vi "main.vi"() -> ()   [LabVIEW 2018]
uses:
  #include/Global_usbComm.vi
  <vilib>/Utility/file.llb/Read Delimited Spreadsheet (string).vi
panel:
  out "negative incline":dbl
  out "tabletType":string
  out "audioType":string
  out "Display":string
  out "TV":string
  out "decimal integer string":string
  out "device":u32
  out "FAN":string
  out "fanType":string
  out "upperLimit":dbl
  out "lowerLimit":dbl
  out "MAX":dbl
  out "upper":dbl
  out "middle":dbl
  out "lower":dbl
  out "minMax":dbl
  out "USB":string
  out "refnum out":refnum<file>
  in  "Tab Control":T1(tab)
  out "Welcome to Console Test":picture
  out "Version":string[][](array[string])
  in  "User Name":string
  out "Console Name":string
  out "Console Number":string
  in  "Work Station":string
  in  "Vendor Name":string
  in  "Vendor Number":string
  in  "EQF1259 com port":refnum<visa-resource-name>
  out "Firmware Reference":string
  out "Initialize Test":string
  out "Config and Fixture Setup":string
  in  "scanSerial":string="387495-JJ02Y101637"
  out "resultSerial":bool
  out "PartNumber":string
  out "COSMETIC-3, 4":string
  in  "Cos0":bool
  in  "Cos1":bool
  in  "Con0":bool
  in  "Con1":bool
  out "FIXTURE_SETUP-1":string
  out "Connection":picture
  out "Voltage":string
  out "Power On":cluster{dbl, dbl}(graph)
  out "Current":string
  out "POWER_UP-5, 6":string
  in  "Pow0":bool
  in  "Pow1":bool
  out "PowerOn":bool
  out "CurrentOn":bool
  out "BLE_SETUP-2":string
  out "BLE_CONNECT-7":string
  in  "BLE1":bool
  in  "BLE0":bool
  in  "Cal1":bool
  in  "Cal0":bool
  in  "Dis1":bool
  in  "Dis0":bool
  in  "key1":bool
  in  "key0":bool
  out "MAINTENANCE MODE-8, 9, 10, 11":string
  in  "Enter Firmware":string
  in  "E-Stop":bool
  out "MPH/KPH":string
  out "PWM":string
  out "FREQUENCY":string
  out "START":string
  out "MID":string
  out "SPEED TREADMILL":dbl(knob) scale=0.0..12.1
  out "MAX":string
  out "Smin":bool=TRUE
  out "Smid":bool=TRUE
  out "Smax":bool=TRUE
  out "PWM_RPM":string
  out "MaxSpeed Time (s)":dbl caption="Elapsed Time (s)"
  out "SPEED AEROBIC":dbl(knob) scale=0.0..25.0
  out "RPM AEROBIC":dbl(knob) scale=0.0..200.0
  in  "Tac0":bool
  in  "Tac1":bool
  in  "RES1":bool
  in  "RES0":bool
  out "overCurrent":bool
  out "RESISTANCE-15":string
  out "RESISTANCE/CURRENT":cluster{dbl, dbl}(graph)
  out "resistance result":bool
  out "ADC hi":bool=TRUE
  out "ADC mid":bool=TRUE
  out "ADC low":bool=TRUE
  out "ADC value":dbl
  out "current#":string
  out "BLE PULSE":u32(graph)
  in  "PUL1":bool
  in  "PUL0":bool
  out "Pulse#":u32
  out "PULSE-17":string
  out "FanCurrent":dbl(graph)
  in  "FAN1":bool
  in  "FAN0":bool
  out "Ifan":string
  out "limitFan":bool
  out "currentMaxFan":string
  out "FAN-18":string
  out "limitAudio":bool
  out "Iaudio":string
  out "AudioCurrent":dbl(graph)
  in  "AUD0":bool
  in  "AUD1":bool
  out "currentMaxAudio":string
  out "AUDIO-19":string
  in  "TV0":bool
  in  "TV1":bool
  out "TVCurrent":dbl(graph)
  out "Itv":string
  out "limitTV":bool
  out "currentMaxTV":string
  out "TV-20":string
  out "limitUSB":bool
  out "Iusb":string
  in  "USB1":bool
  in  "USB0":bool
  out "currentMaxUSB":string
  out "USBCurrent":dbl(graph)
  out "USB-16":string
  out "resultIncline":bool
  out "INCLINE":dbl(graph)
  in  "E-Stop/Incline":bool
  out "INCLINE-14":string
  out "inclineMax":dbl
  out "inclineMin":dbl
  out "inclineMid":dbl
  out "Imin":bool=TRUE
  out "Imid":bool=TRUE
  out "Imax":bool=TRUE
  out "Incline Time (s)":dbl caption="Elapsed Time (s)"
  out "limitCSafe":bool
  out "Icsafe":string
  in  "CSA1":bool
  in  "CSA0":bool
  out "currentMaxCSafe":string
  out "CSafeCurrent":dbl(graph)
  out "CSAFE-21":string
  out "limitWahoo":bool
  out "Iwahoo":string
  in  "WAH1":bool
  in  "WAH0":bool
  out "currentMaxWahoo":string
  out "WahooCurrent":dbl(graph)
  out "WAHOO-22":string
  in  "ANO0":bool
  in  "ANO1":bool
  out "Another":picture
  out "Failed":picture
  out "Test Log":string
  out "# of Failed Samples":i32
  out "# of Samples":i32
  out "Goodbye!":picture
  # "Scan Console Serial Number"
  # "Does Cosmetic Pass Inspection?"
  # "Is the console connected correctly?"
  # "Did Console Power ON?"
  # "Calibrate?"
  # "Display?"
  # "Keys?"
  # "Does Max Speed/RPM On Console Match Indicator?"
  # "Did Resistance Reach Max?"
  # "Does The Pulse# Match The Display?"
  # "Did The Fan Function Well?"
  # "Does Incline On Console Change?"
  # "Would You Like To Test Another Console?"
  # "Console Failed Test!"
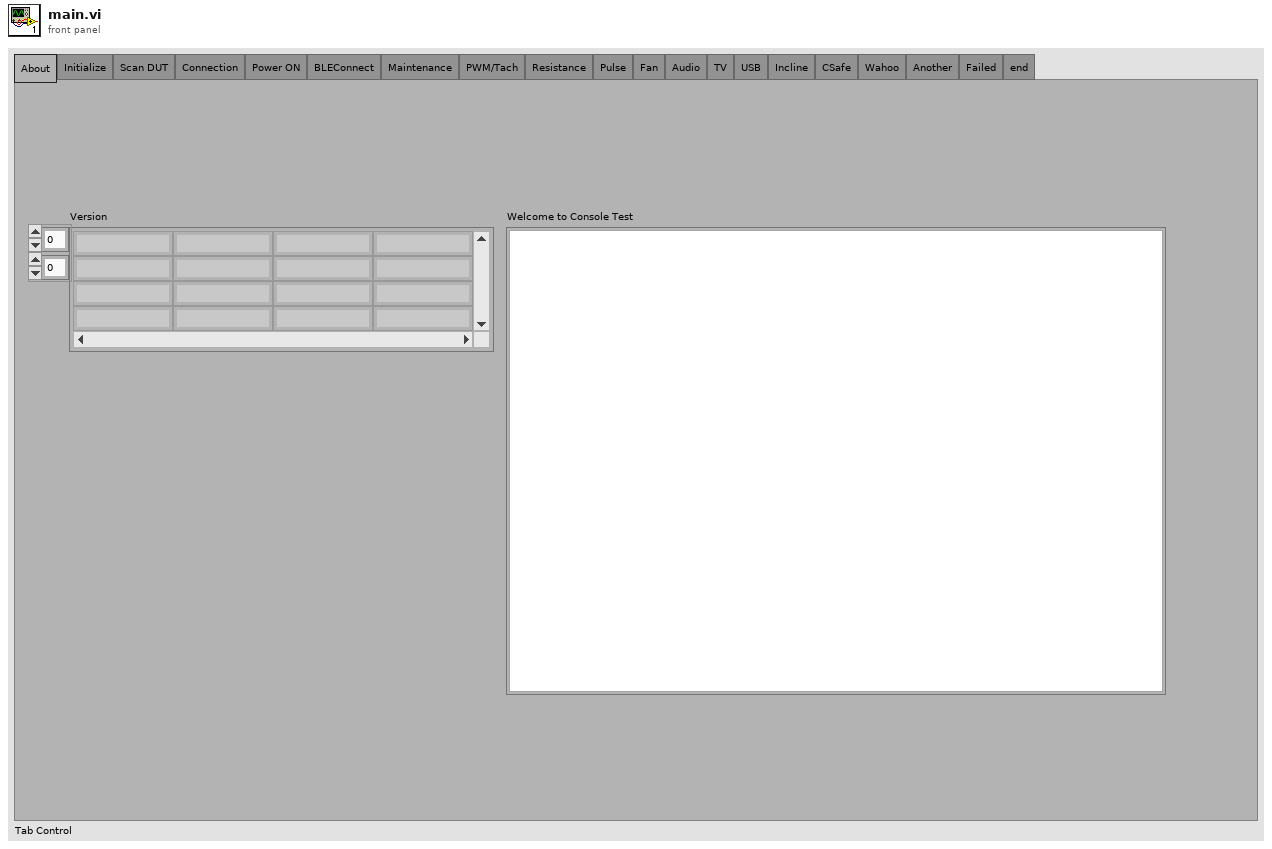
[diagram p1: front panel]
types:
  T1 = enum32{"About", "Initialize", "Scan DUT", "Connection", "Power ON", "BLEConnect", "Maintenance", "PWM/Tach", "Resistance", "Pulse", "Fan", "Audio", "TV", "USB", "Incline", "CSafe", "Wahoo", "Another", "Failed", "end"}
  T2 = enum16{"name", "number", "type", "ctlr/pwrbrd", "firmware", "mcu", "display"}
  T3 = enum16{"User", "Station", "Vendor", "Number", "Record"}
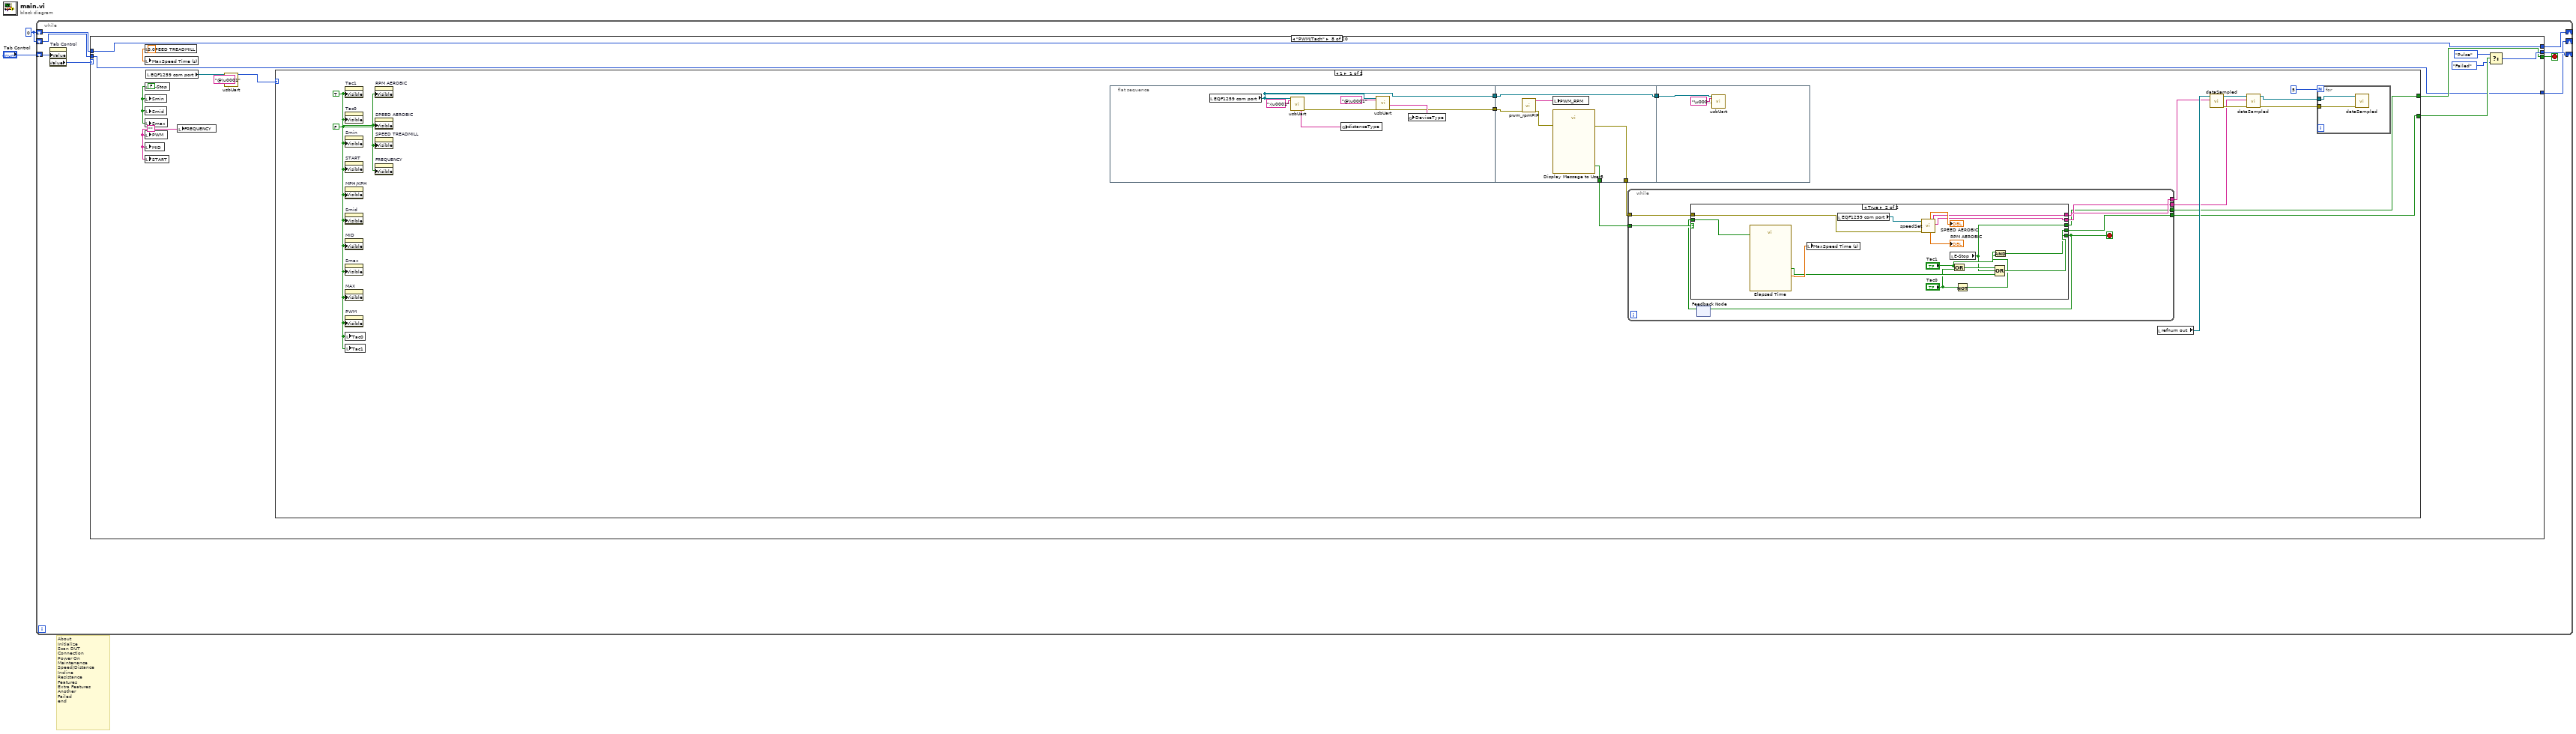
[diagram p0: block diagram]
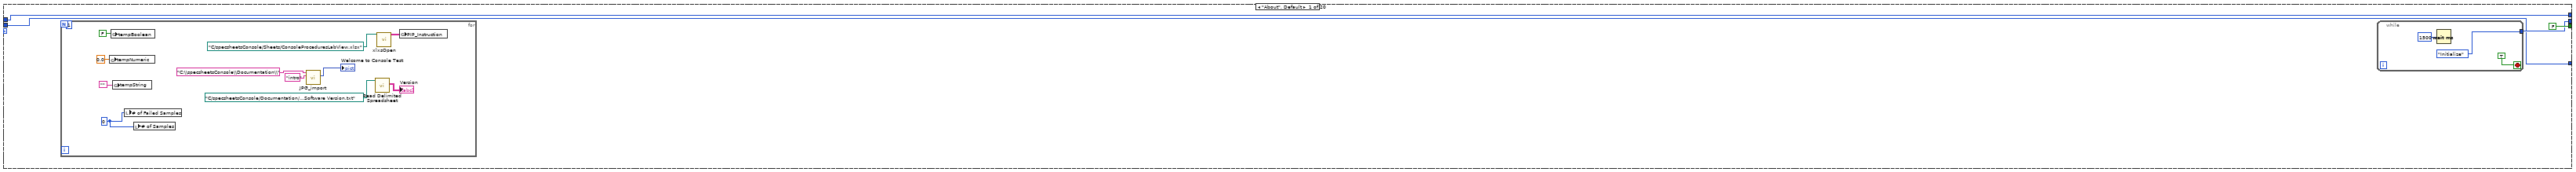
[diagram p2: hidden frame]
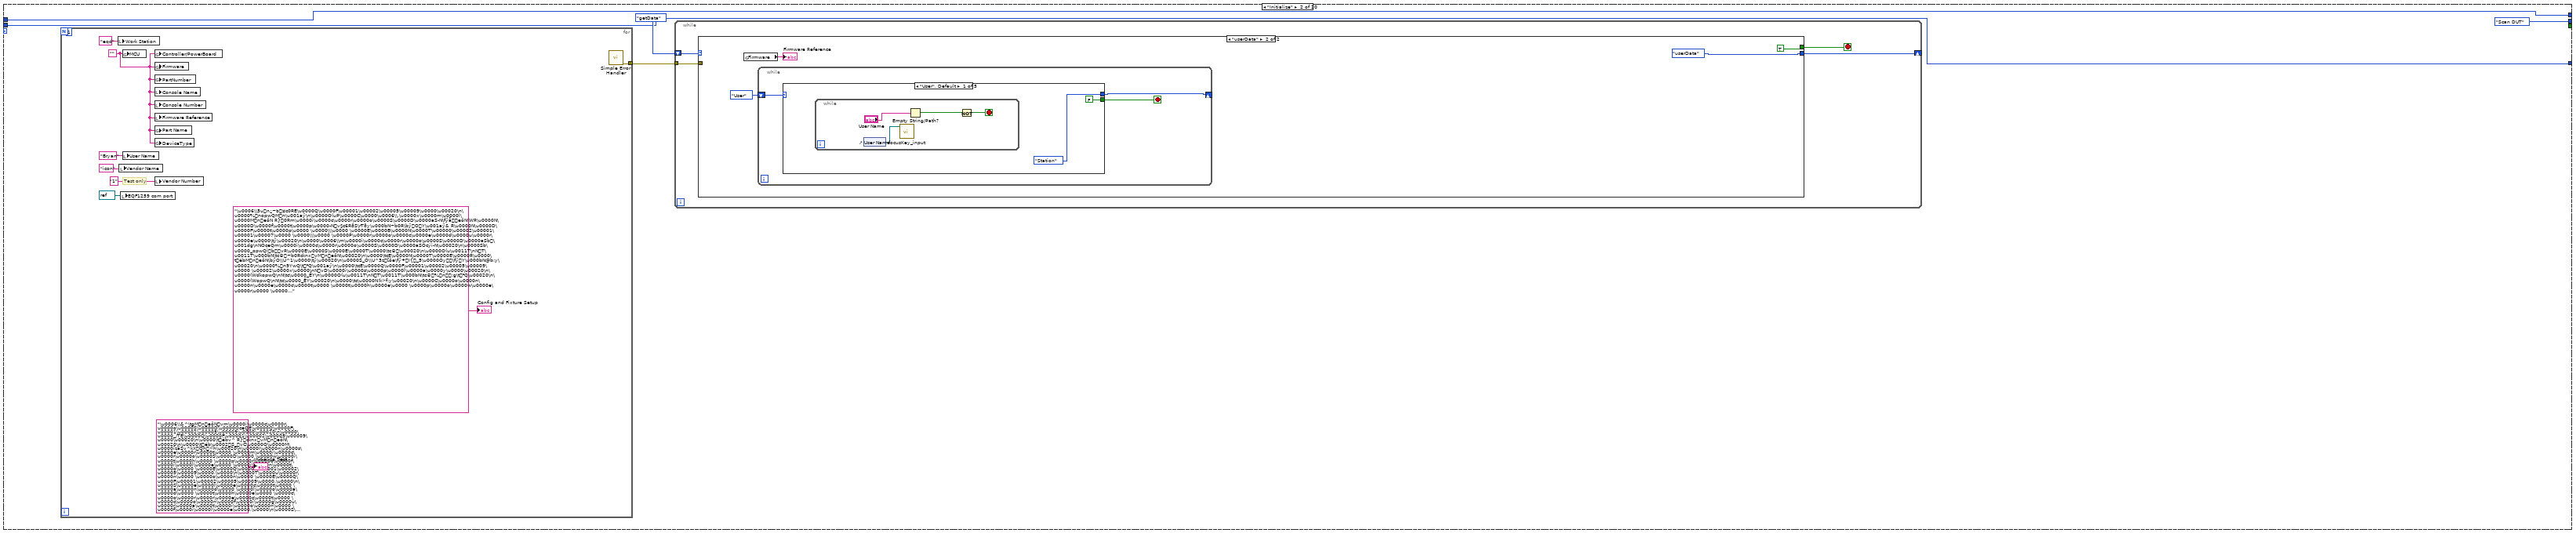
[diagram p3: hidden frame]
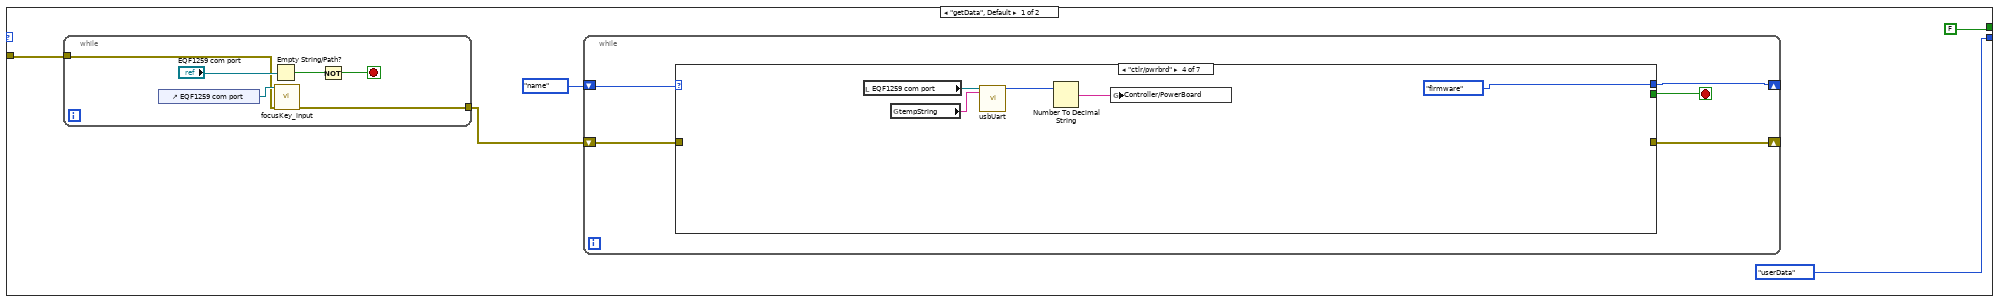
[diagram p4: hidden frame]
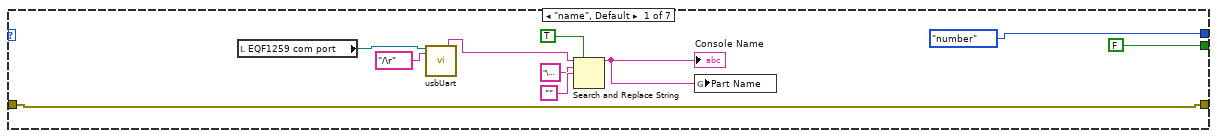
[diagram p5: hidden frame]
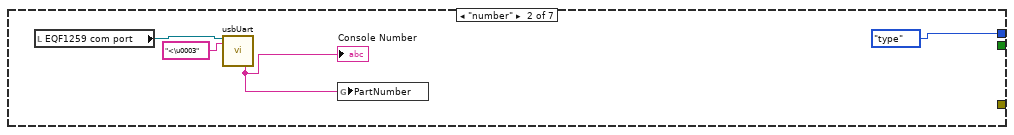
[diagram p6: hidden frame]
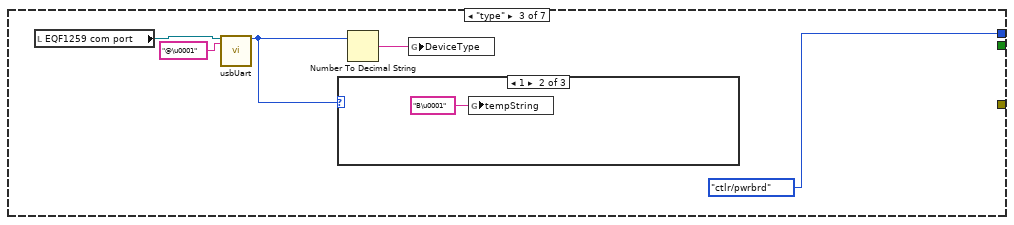
[diagram p7: hidden frame]
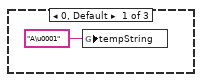
[diagram p8: hidden frame]
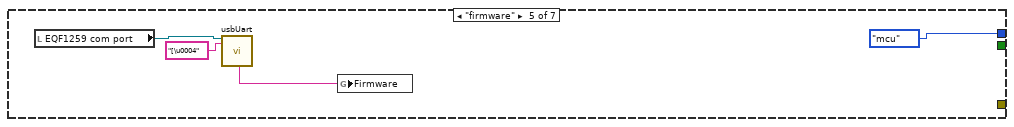
[diagram p10: hidden frame]
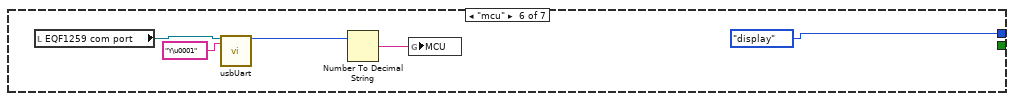
[diagram p11: hidden frame]
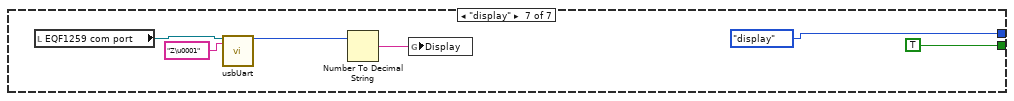
[diagram p12: hidden frame]
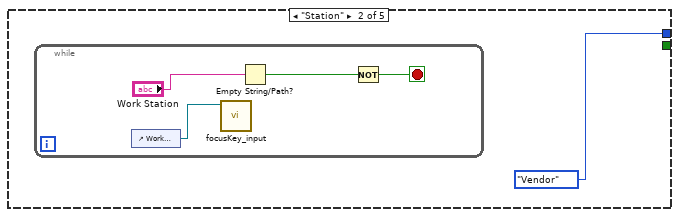
[diagram p13: hidden frame]
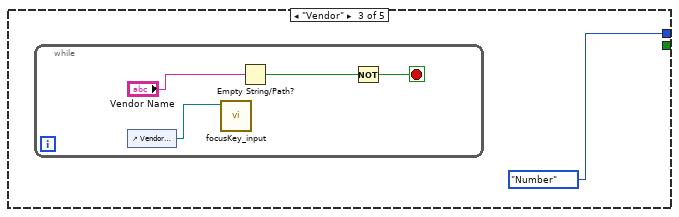
[diagram p14: hidden frame]
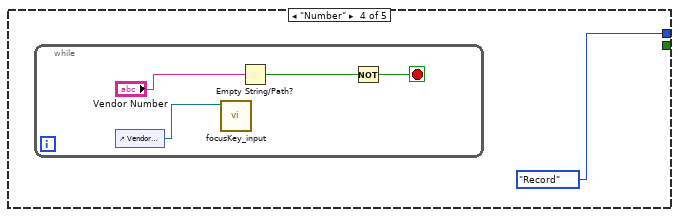
[diagram p15: hidden frame]
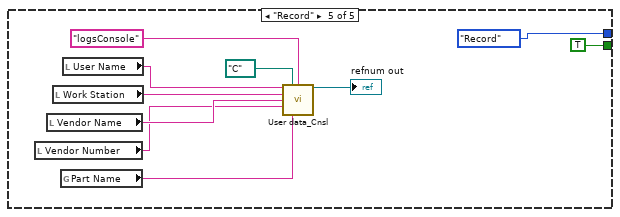
[diagram p16: hidden frame]
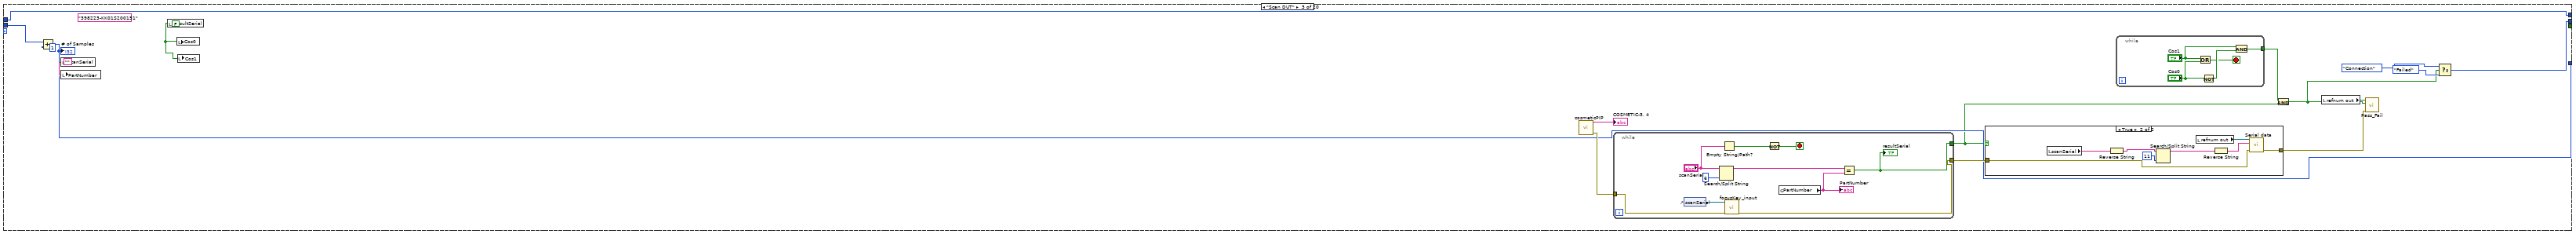
[diagram p17: hidden frame]
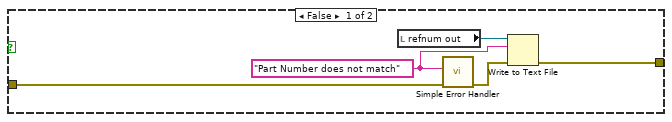
[diagram p18: hidden frame]
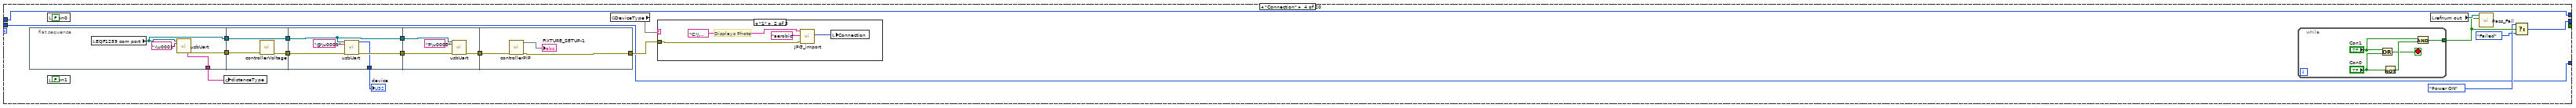
[diagram p19: hidden frame]
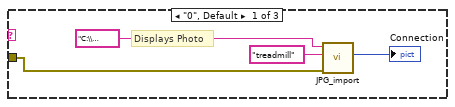
[diagram p20: hidden frame]
diagram:
  w1 = 0
  # "About\nInitialize\nScan DUT\nConnection\nPower On\nMaintenance\nSpeed/Distance\nIncline\nResistance\nFeatures\nExtra Features\nAnother\nFailed\nend"
  n1 = while {
    shift-right: [w9] -> _
    shift-left: "Tab Control" -> [w8]
    shift-right: [w4] -> _
    shift-left: w1 -> [w6]
    shift-right: [w3] -> _
    shift-left: w1 -> [w5]
    stop <- w10 stop-if-true
    n2 = property on="Tab Control" class="TabCtl (strict)"("Value"=w8) -> ("Value"=w7:T1)  [unwired: 2 in, 2 out]
    n3 = case shown="\"PWM/Tach\"" w7 {
      tunnel: [FALSE _ _ _ _ _ _ w444 w643 _ _ _ _ _ _ _ _ _ _ TRUE] -> w10
      tunnel: [w13 T1."Scan DUT" ("Tab Control") w152 w200 w258 w327 w363 w446 w645 w765 w901 w941 w1023 w1051 w1151 w1228 w1288 w1347 T1."Another" ("Tab Control") T1."end" ("Tab Control")] -> w9
      tunnel: w6 -> [w12 w31 w150 w190 w246 w323 w356 w435 w639 w756 w890 w922 w1000 w1043 w1140 w1218 w1277 w1336 w1354 w1368]
      tunnel: w5 -> [w11 w30 w148 w189 w245 w322 w355 w434 w638 w755 w889 w921 w999 w1042 w1139 w1217 w1276 w1335 w1356 w1367]
      tunnel: [w12 w31 w149 w190 w246 w323 w356 w435 w639 w756 w890 w922 w1000 w1043 w1140 w1218 w1277 w1336 w1354 w1368] -> w4
      tunnel: [w11 w30 w148 w189 w245 w322 w355 w434 w638 w755 w889 w921 w999 w1042 w1139 w1217 w1276 w1335 w1355 w1367] -> w3
      frame "About", Default {
        n4 = for {
          N: 1 -> [_]
          w16 = 0
          n5 = global write "Global_usbComm.vi" "tempNumeric"(0.0 ("tempNumeric")) -> ()
          n6 = global write "Global_usbComm.vi" "tempBoolean"(FALSE) -> ()
          n7 = global write "Global_usbComm.vi" "tempString"("" ("tempString")) -> ()
          n8 = local write "# of Failed Samples"(w16) -> ()
          n9 = local write "# of Samples"(w16) -> ()
          n10 = call "JPG_import.vi"("File name"="intro" ("Complete File path"), "File path"="C:\\specsheetsConsole\\Documentation\\" ("File name")) -> ("new picture"=→"Welcome to Console Test":picture)  [unwired: 7 in, 2 out]
          n11 = call-poly <vilib>:"Read Delimited Spreadsheet.vi"("file path (dialog if empty)"=path "C:/specsheetsConsole/Documentation/...Software Version.txt") -> ("all rows"=→"Version":string[][])  [unwired: 9 in, 5 out]
          n12 = call "xlxsOpen.vi"("PIP Instruction Path"=path "C:/specsheetsConsole/Sheets/ConsoleProceduresLabView.xlsx") -> ("Shared_strings"=w25:string[][])  [unwired: 10 in, 4 out]
          n13 = global write "Global_usbComm.vi" "PIP_Instruction"(w25) -> ()
        }
        n14 = while {
          tunnel: [T1."Initialize" ("Tab Control")] -> w13
          stop <- TRUE stop-if-true
          n15 = Wait (ms)(milliseconds to wait=u32 1500) -> ()  [unwired: 1 out]
        }
      }
      frame "Initialize" {
        n16 = for {
          N: 1 -> [_]
          tunnel: [w37] -> w33
          w43 = ""
          # "Test only"
          n17 = local write "Work Station"("eqd" ("Work Station")) -> ()
          n18 = local write "Vendor Name"("icon" ("Vendor Name")) -> ()
          n19 = local write "EQF1259 com port"(refnum<visa-resource-name> refnum ("VISA resource name")) -> ()
          n20 = global write "Global_usbComm.vi" "MCU"(w43) -> ()
          n21 = local write "User Name"("Bryan" ("User Name")) -> ()
          n22 = global write "Global_usbComm.vi" "Controller/PowerBoard"(w43) -> ()
          n23 = global write "Global_usbComm.vi" "Firmware"(w43) -> ()
          n24 = global write "Global_usbComm.vi" "PartNumber"(w43) -> ()
          n25 = local write "Console Name"(w43) -> ()
          n26 = local write "Console Number"(w43) -> ()
          n27 = local write "Firmware Reference"(w43) -> ()
          n28 = global write "Global_usbComm.vi" "Part Name"(w43) -> ()
          n29 = global write "Global_usbComm.vi" "DeviceType"(w43) -> ()
          n30 = local write "Vendor Number"("1" ("Vendor Number")) -> ()
          n31 = call <vilib>:"Simple Error Handler.vi"() -> ("error out"=w37:errorcluster)  [unwired: 5 in, 4 out]
          "Initialize Test" <- "\u0006\\&^\tgMneöNvm\u0000i\u0000c\u0000r\u0000o\u0000S\u0000D\u0000ÒceQE\u0000Q\u0000F\u00001\u00002\u00005\u00009\u0000\u00020\n\u0000\u0000_/TE\u0000Q\u0000F\u00001\u00002\u00005\u00009\u0000\u00020\n\u0000\tébv^ R}cknxvMneöN\u00020\n\u0000\téb\u0002S_vC\u0000O\u0000M\u0000ïzãSv^kXQh<h\u00020\n\u0000I\u0000n\u0000s\u0000e\u0000r\u0000t\u0000 \u0000m\u0000i\u0000c\u0000r\u0000o\u0000S\u0000D\u0000 \u0000w\u0000i\u0000t\u0000h\u0000 \u0000p\u0000r\u0000o\u0000f\u0000i\u0000l\u0000e\u0000 \u0000i\u0000n\u0000t\u0000o\u0000 \u0000E\u0000Q\u0000F\u00001\u00002\u00005\u00009\u0000.\u0000\n\u0000T\u0000u\u0000r\u0000n\u0000 \u0000o\u0000n\u0000 \u0000E\u0000Q\u0000F\u00001\u00002\u00005\u00009\u0000.\u0000\n\u0000S\u0000e\u0000l\u0000e\u0000c\u0000t\u0000 \u0000a\u0000n\u0000d\u0000 \u0000l\u0000o\u0000a\u0000d\u0000 \u0000t\u0000h\u0000e\u0000 \u0000c\u0000o\u0000r\u0000r\u0000e\u0000c\u0000t\u0000 \u0000c\u0000o\u0000n\u0000f\u0000i\u0000g\u0000u\u0000r\u0000a\u0000t\u0000i\u0000o\u0000n\u0000 \u0000f\u0000i\u0000l\u0000e\u0000.\u0000\n\u0000S\u0000e\u0000l\u0000e\u0000c\u0000t\u0000 \u0000t\u0000h\u0000e\u0000 \u0000p\u0000r\u0000o\u0000p\u0000e\u0000r\u0000 \u0000c\u0000o\u0000m\u0000 \u0000p\u0000o\u0000r\u0000t\u0000 \u0000a\u0000n\u0000d\u0000 \u0000c\u0000o\u0000m\u0000p\u0000l\u0000e\u0000t\u0000e\u0000 \u0000t\u0000h\u0000e\u0000 \u0000f\u0000o\u0000r\u0000m\u0000.\u0000"
          "Config and Fixture Setup" <- "\u0006\\5un¿~Þ¥c0RE\u0000Q\u0000F\u00001\u00002\u00005\u00009\u0000\u00020\n\u0000¾nopwQMn\u001aÿ\n\u0000O(uP\u0000C\u0000\u0006\\.\u0000x\u0000m\u0000l\u0000MneöN R}0Rm\u0000i\u0000c\u0000r\u0000o\u0000S\u0000D\u0000aS-N\fÿåeöN(WR\u0000N\u0000D\u0000f\u0000t\u0000p\u0000-Nv§c6RðS\rTðy\u000bN~b0R\bÿOY\u001aÿ& R\u0000N\u0000D\u0000F\u0000t\u0000p\u0000 \u0000\\\u0000 \u0000E\u0000B\u0000N\u0000T\u00000\u00002\u00001\u00001\u00007\u0000 \u0000\\\u0000 \u0000P\u0000r\u0000o\u0000c\u0000e\u0000d\u0000u\u0000r\u0000e\u0000\tÿ\u00020\n\u0000\u0006\\m\u0000i\u0000c\u0000r\u0000o\u0000S\u0000D\u0000aSb\u001dg\nNÒceQm\u0000i\u0000c\u0000r\u0000o\u0000S\u0000D\u0000aSÒcýi-N\u00020\n\u0000Sb\u0000_opwQÌbvR\u0000E\u0000S\u0000E\u0000T\u0000\tc®\u00020\n\u0000O(u\u0011T\nNT\u0011T\u000bN\tc®~b0RcknxvMneöN\u00020\n\u0000\tcE\u0000N\u0000T\u0000E\u0000R\u0000\tébMneöN\bÿO\\U^1\u0000\tÿ\u00020\n\u0000S_O\\U^3z[öe\fÿ÷I{_5\u0000Òy\fÿY\u000bN@b:y\u00020\n\u0000¾n9YwQ\t²Q\u001aÿ\n\u0000\tcE\u0000Q\u0000F\u00001\u00002\u00005\u00009\u0000 \u00002\u0000x\u0000\nNvD\u0000i\u0000s\u0000p\u0000l\u0000a\u0000y\u0000\u00020\n\u0000(WdkopwQ\nN\tc\u0000_ËY\n\u0000O(u\u0011T\nNT\u0011T\u000bN\tc®¾n:g\t²Q\u00020\n\u0000(WopwQ\nN\tc\u0000_ËY\u00020\n\u0000\tc\u0000N!k>f:y\u00020\n\u0000C\u0000o\u0000n\u0000n\u0000e\u0000c\u0000t\u0000 \u0000t\u0000h\u0000e\u0000 \u0000p\u0000o\u0000w\u0000e\u0000r\u0000 \u0000..."
        }
        n32 = while {
          shift-right: [w46] -> _
          shift-left: enum16{"getData", "userData"}."getData" -> [w48]
          tunnel: w33 -> [w45]
          stop <- w47 stop-if-true
          n33 = case shown="\"userData\"" w48 {
            tunnel: [FALSE TRUE] -> w47
            tunnel: [enum16{"getData", "userData"}."userData" enum16{"getData", "userData"}."userData"] -> w46
            tunnel: w45 -> [w49 _]
            frame "getData", Default {
              n34 = while {
                tunnel: [w55] -> w51
                tunnel: w49 -> [w54]
                stop <- w56 stop-if-true
                n35 = control-ref of="EQF1259 com port"() -> (w59:refnum<vi>)
                n36 = Empty String/Path?(string/path="EQF1259 com port") -> (empty?=w57:bool)
                n37 = call "focusKey_input.vi"("error in (no error)"=w54, "reference"=w59) -> ("error out"=w55:errorcluster)  [unwired: 9 in]
                n38 = Not(x=w57) -> (.not. x?=w56:bool)
              }
              n39 = while {
                shift-right: [w60] -> _
                shift-left: T2."name" -> [w64]
                shift-right: [w61] -> _
                shift-left: w51 -> [w62]
                stop <- w63 stop-if-true
                n40 = case shown="\"ctlr/pwrbrd\"" w64 {
                  tunnel: [FALSE _ _ _ _ _ TRUE] -> w63
                  tunnel: w62 -> [w71 _ _ _ _ _ _]
                  tunnel: [T2."number" T2."type" T2."ctlr/pwrbrd" T2."firmware" T2."mcu" T2."display" T2."display"] -> w60
                  tunnel: [w71 _ _ _ _ _ _] -> w61
                  frame "name", Default {
                    n41 = local read "EQF1259 com port"() -> (w72:refnum<visa-resource-name>)
                    n42 = call "usbUart.vi"("VISA resource name"=w72, "write buffer"="/\r" ("write buffer buffer")) -> ("valid byte"=w69:string)  [unwired: 2 in, 15 out]
                    n43 = Search and Replace String(replace all?=TRUE ("replace all? (F)"), input string=w69, search string="\u0000", replace string="") -> (result string=w66:string)  [unwired: 4 in, 3 out]
                    "Console Name" <- w66
                    n44 = global write "Global_usbComm.vi" "Part Name"(w66) -> ()
                  }
                  frame "number" {
                    n45 = local read "EQF1259 com port"() -> (w77:refnum<visa-resource-name>)
                    n46 = call "usbUart.vi"("VISA resource name"=w77, "write buffer"="<\u0003" ("write buffer buffer")) -> ("PartNumber"=w76:string)  [unwired: 2 in, 15 out]
                    "Console Number" <- w76
                    n47 = global write "Global_usbComm.vi" "PartNumber"(w76) -> ()
                  }
                  frame "type" {
                    n48 = local read "EQF1259 com port"() -> (w82:refnum<visa-resource-name>)
                    n49 = call "usbUart.vi"("VISA resource name"=w82, "write buffer"="@\u0001" ("write buffer buffer")) -> ("number[0]"=w81:u32)  [unwired: 2 in, 15 out]
                    n50 = case shown="1" w81 {
                      frame 0, Default {
                        n51 = global write "Global_usbComm.vi" "tempString"("A\u0001" ("write buffer buffer")) -> ()
                      }
                      frame 1 {
                        n52 = global write "Global_usbComm.vi" "tempString"("B\u0001" ("write buffer")) -> ()
                      }
                      frame 3 {
                        # "Rower_Basic"
                      }
                    }
                    n53 = Number To Decimal String(number=w81) -> (decimal integer string=w80:string)  [unwired: 1 in]
                    n54 = global write "Global_usbComm.vi" "DeviceType"(w80) -> ()
                  }
                  frame "ctlr/pwrbrd" {
                    n55 = local read "EQF1259 com port"() -> (w90:refnum<visa-resource-name>)
                    n56 = global read "Global_usbComm.vi" "tempString"() -> (w87:string)
                    n57 = call "usbUart.vi"("VISA resource name"=w90, "write buffer"=w87) -> ("number[0]"=w89:u32)  [unwired: 2 in, 15 out]
                    n58 = Number To Decimal String(number=w89) -> (decimal integer string=w88:string)  [unwired: 1 in]
                    n59 = global write "Global_usbComm.vi" "Controller/PowerBoard"(w88) -> ()
                  }
                  frame "firmware" {
                    n60 = local read "EQF1259 com port"() -> (w94:refnum<visa-resource-name>)
                    n61 = call "usbUart.vi"("VISA resource name"=w94, "write buffer"="[\u0004") -> ("BB FW"=w92:string)  [unwired: 2 in, 15 out]
                    n62 = global write "Global_usbComm.vi" "Firmware"(w92) -> ()
                  }
                  frame "mcu" {
                    n63 = local read "EQF1259 com port"() -> (w97:refnum<visa-resource-name>)
                    n64 = call "usbUart.vi"("VISA resource name"=w97, "write buffer"="Y\u0001") -> ("number[0]"=w99:u32)  [unwired: 2 in, 15 out]
                    n65 = Number To Decimal String(number=w99) -> (decimal integer string=w96:string)  [unwired: 1 in]
                    n66 = global write "Global_usbComm.vi" "MCU"(w96) -> ()
                  }
                  frame "display" {
                    n67 = local read "EQF1259 com port"() -> (w102:refnum<visa-resource-name>)
                    n68 = call "usbUart.vi"("VISA resource name"=w102, "write buffer"="Z\u0001") -> ("number[0]"=w105:u32)  [unwired: 2 in, 15 out]
                    n69 = Number To Decimal String(number=w105) -> (decimal integer string=w103:string)  [unwired: 1 in]
                    n70 = global write "Global_usbComm.vi" "Display"(w103) -> ()
                  }
                }
              }
            }
            frame "userData" {
              n71 = global read "Global_usbComm.vi" "Firmware"() -> (→"Firmware Reference":string)
              n72 = while {
                shift-right: [w110] -> _
                shift-left: T3."User" -> [w112]
                stop <- w111 stop-if-true
                n73 = case shown="\"User\", Default" w112 {
                  tunnel: [FALSE _ _ _ TRUE] -> w111
                  tunnel: [T3."Station" T3."Vendor" T3."Number" T3."Record" T3."Record"] -> w110
                  frame "User", Default {
                    n74 = while {
                      stop <- w116 stop-if-true
                      n75 = control-ref of="User Name"() -> (w115:refnum<vi>)
                      n76 = call "focusKey_input.vi"("reference"=w115) -> ()  [unwired: 10 in, 1 out]
                      n77 = Empty String/Path?(string/path="User Name") -> (empty?=w118:bool)
                      n78 = Not(x=w118) -> (.not. x?=w116:bool)
                    }
                  }
                  frame "Station" {
                    n79 = while {
                      stop <- w121 stop-if-true
                      n80 = control-ref of="Work Station"() -> (w120:refnum<vi>)
                      n81 = call "focusKey_input.vi"("reference"=w120) -> ()  [unwired: 10 in, 1 out]
                      n82 = Empty String/Path?(string/path="Work Station") -> (empty?=w123:bool)
                      n83 = Not(x=w123) -> (.not. x?=w121:bool)
                    }
                  }
                  frame "Vendor" {
                    n84 = while {
                      stop <- w126 stop-if-true
                      n85 = control-ref of="Vendor Name"() -> (w125:refnum<vi>)
                      n86 = call "focusKey_input.vi"("reference"=w125) -> ()  [unwired: 10 in, 1 out]
                      n87 = Empty String/Path?(string/path="Vendor Name") -> (empty?=w128:bool)
                      n88 = Not(x=w128) -> (.not. x?=w126:bool)
                    }
                  }
                  frame "Number" {
                    n89 = while {
                      stop <- w131 stop-if-true
                      n90 = control-ref of="Vendor Number"() -> (w130:refnum<vi>)
                      n91 = call "focusKey_input.vi"("reference"=w130) -> ()  [unwired: 10 in, 1 out]
                      n92 = Empty String/Path?(string/path="Vendor Number") -> (empty?=w133:bool)
                      n93 = Not(x=w133) -> (.not. x?=w131:bool)
                    }
                  }
                  frame "Record" {
                    n94 = local read "Vendor Number"() -> (w137:string)
                    n95 = local read "Vendor Name"() -> (w140:string)
                    n96 = local read "Work Station"() -> (w141:string)
                    n97 = global read "Global_usbComm.vi" "Part Name"() -> (w136:string)
                    n98 = local read "User Name"() -> (w142:string)
                    n99 = call "User data_Cnsl.vi"("Inspector"=w142, "base path"=path "C:/", "prompt (Create Folder)"="logsConsole", "Station"=w141, "Vendor"=w140, "Number"=w137, "file name"=w136) -> ("refnum out"=→"refnum out":refnum<file>)  [unwired: 7 in, 1 out]
                  }
                }
              }
            }
          }
        }
      }
      frame "Scan DUT" {
        (unwired) "398223-KK01S200151"
        w144 = FALSE
        w155 = ""
        n100 = Add(x=w150, y=1) -> (x+y=w149:i32)
        "# of Samples" <- w149
        n101 = local write "scanSerial"(w155) -> ()
        n102 = local write "PartNumber"(w155) -> ()
        n103 = local write "resultSerial"(w144) -> ()
        n104 = local write "Cos0"(w144) -> ()
        n105 = local write "Cos1"(w144) -> ()
        n106 = call "cosmeticPIP.vi"() -> ("error out"=w156:errorcluster, "COSMETIC-3, 4"=→"COSMETIC-3, 4":string)  [unwired: 10 in]
        n107 = while {
          tunnel: [w186] -> w160
          tunnel: [w180] -> w145
          tunnel: w156 -> [w179]
          stop <- w187 stop-if-true
          n108 = control-ref of="scanSerial"() -> (w185:refnum<vi>)
          n109 = Search/Split String(string="scanSerial", offset (0)=6) -> (substring before match=w184:string)  [unwired: 1 in, 2 out]
          n110 = Empty String/Path?(string/path="scanSerial") -> (empty?=w188:bool)
          n111 = call "focusKey_input.vi"("error in (no error)"=w179, "reference"=w185) -> ("error out"=w186:errorcluster)  [unwired: 9 in]
          n112 = Not(x=w188) -> (.not. x?=w187:bool)
          n113 = global read "Global_usbComm.vi" "PartNumber"() -> (w183:string)
          "PartNumber" <- w183
          n114 = Equal?(x=w184, y=w183) -> (x = y?=w180:bool)
          "resultSerial" <- w180
        }
        n115 = case shown="True" w145 {
          tunnel: w160 -> [w166 w171]
          tunnel: [w167 w172] -> w158
          frame False {
            w169 = "Part Number does not match" ("error source (\" \")")
            n116 = local read "refnum out"() -> (w168:refnum<file>)
            n117 = call <vilib>:"Simple Error Handler.vi"("error source (\" \")"=w169, "error in (no error)"=w166) -> ("error out"=w170:errorcluster)  [unwired: 3 in, 4 out]
            n118 = Write to Text File(file (use dialog)=w168, text=w169, error in=w170) -> (error out=w167:errorcluster)  [unwired: 1 in, 2 out]
          }
          frame True {
            n119 = local read "scanSerial"() -> (w175:string)
            n120 = Reverse String(1:w175) -> (0:w177:string)
            n121 = Search/Split String(string=w177, offset (0)=11) -> (substring before match=w178:string)  [unwired: 1 in, 2 out]
            n122 = local read "refnum out"() -> (w173:refnum<file>)
            n123 = Reverse String(1:w178) -> (0:w174:string)
            n124 = call "Serial data.vi"("error in"=w171, "Serial Number"=w174, "refnum in"=w173) -> ("error out"=w172:errorcluster)  [unwired: 7 in, 1 out]
          }
        }
        n125 = while {
          tunnel: [w161] -> w146
          stop <- w164 stop-if-true
          n126 = Or(x="Cos1", y="Cos0") -> (x .or. y?=w164:bool)
          n127 = Not(x="Cos0") -> (.not. x?=w165:bool)
          n128 = And(x="Cos1", y=w165) -> (x .and. y?=w161:bool)
        }
        n129 = And(x=w146, y=w145) -> (x .and. y?=w147:bool)
        n130 = local read "refnum out"() -> (w159:refnum<file>)
        n131 = call "Pass_Fail.vi"("error in (no error)"=w158, "OK"=w147, "Byte Stream File in"=w159) -> ()  [unwired: 7 in, 2 out]
        n132 = Select(t=T1."Connection" ("Tab Control"), s=w147, f=T1."Failed" ("Tab Control")) -> (s? t:f=w152:T1)
      }
      frame "Connection" {
        n133 = flat-sequence {
          tunnel: [w211] -> w204
          tunnel: [w210] -> w199
          tunnel: [w209] -> w197
          tunnel: w199 -> [w214]
          tunnel: [w213] -> w198
          tunnel: w197 -> [w215]
          tunnel: [w215] -> w196
          tunnel: w198 -> [w219]
          tunnel: w196 -> [w217]
          tunnel: [w218] -> w194
          tunnel: [w217] -> w192
          tunnel: [w216] -> w191
          tunnel: w194 -> [w224]
          tunnel: [w223] -> w193
          tunnel: w192 -> [w222]
          tunnel: w193 -> [w226]
          tunnel: [w225] -> w195
          frame #0 {
            n134 = local read "EQF1259 com port"() -> (w209:refnum<visa-resource-name>)
            n135 = call "usbUart.vi"("VISA resource name"=w209, "write buffer"="›\u0001") -> ("PartNumber"=w211:string, "error out"=w210:errorcluster)  [unwired: 2 in, 14 out]
          }
          frame #1 {
            n136 = call "controllerVoltage.vi"("error in (no error)"=w214) -> ("error out"=w213:errorcluster)  [unwired: 10 in]
          }
          frame #2 {
            n137 = call "usbUart.vi"("VISA resource name"=w217, "write buffer"="@\u0001", "error in (no error)"=w219) -> ("number[0]"=w216:u32, "error out"=w218:errorcluster)  [unwired: 1 in, 14 out]
          }
          frame #3 {
            n138 = call "usbUart.vi"("VISA resource name"=w222, "write buffer"="P\u0002", "error in (no error)"=w224) -> ("error out"=w223:errorcluster)  [unwired: 1 in, 15 out]
          }
          frame #4 {
            n139 = call "controllerPIP.vi"("error in (no error)"=w226) -> ("error out"=w225:errorcluster, 3:→"FIXTURE_SETUP-1")  [unwired: 9 in]
          }
        }
        n140 = local write "Con0"(FALSE) -> ()
        n141 = local write "Con1"(FALSE) -> ()
        n142 = global write "Global_usbComm.vi" "distanceType"(w204) -> ()
        n143 = global read "Global_usbComm.vi" "DeviceType"() -> (w203)
        n144 = case shown="\"1\"" w203 {
          tunnel: w195 -> [w228 w235 w236]
          frame "0", Default {
            # "Displays Photo"
            n145 = call "JPG_import.vi"("error in (no error)"=w228, "File name"="treadmill", "File path"="C:\\specsheetsConsole\\Documentation\\" ("File name")) -> ("new picture"=→"Connection":picture)  [unwired: 6 in, 2 out]
          }
          frame "1" {
            # "Displays Photo"
            n146 = call "JPG_import.vi"("error in (no error)"=w235, "File name"="aerobic", "File path"="C:\\specsheetsConsole\\Documentation\\" ("File name")) -> ("new picture"=w232:picture)  [unwired: 6 in, 2 out]
            n147 = local write "Connection"(w232) -> ()
          }
          frame "2" {
            # "Displays Photo"
            n148 = call "JPG_import.vi"("error in (no error)"=w236, "File name"="aerobic", "File path"="C:\\specsheetsConsole\\Documentation\\" ("File name")) -> ("new picture"=w237:picture)  [unwired: 6 in, 2 out]
            n149 = local write "Connection"(w237) -> ()
          }
        }
        n150 = while {
          tunnel: [w240] -> w207
          stop <- w243 stop-if-true
          n151 = Or(x="Con1", y="Con0") -> (x .or. y?=w243:bool)
          n152 = Not(x="Con0") -> (.not. x?=w244:bool)
          n153 = And(x="Con1", y=w244) -> (x .and. y?=w240:bool)
        }
        n154 = local read "refnum out"() -> (w208:refnum<file>)
        n155 = call "Pass_Fail.vi"("OK"=w207, "Byte Stream File in"=w208) -> ()  [unwired: 8 in, 2 out]
        n156 = Select(t=T1."Power ON" ("Tab Control"), s=w207, f=T1."Failed" ("Tab Control")) -> (s? t:f=w200:T1)
        "device" <- w191
      }
      frame "Power ON" {
        w253 = FALSE
        w256 = ""
        n157 = local write "Pow1"(w253) -> ()
        n158 = local write "Pow0"(w253) -> ()
        n159 = property on="Power On" class="WFChart (strict)"("History Data"=cluster{dbl, dbl}[] []) -> ()  [unwired: 2 in, 2 out]
        n160 = local write "Voltage"(w256) -> ()
        n161 = local write "Current"(w256) -> ()
        n162 = global read "Global_usbComm.vi" "POWER_UP-5, 6"() -> (→"POWER_UP-5, 6":string)
        n163 = local write "PowerOn"(w253) -> ()
        n164 = local read "EQF1259 com port"() -> (w248:refnum<visa-resource-name>)
        n165 = call "Display Message to User4"() -> ("error out"=w250:errorcluster)  [unwired: 10 in, 1 out]
        n166 = call "usbUart.vi"("VISA resource name"=w248, "write buffer"="(\u0002", "error in (no error)"=w250) -> ("error out"=w247:errorcluster)  [unwired: 1 in, 15 out]
        n167 = while {
          tunnel: [w279] -> w261
          tunnel: [w284] -> w260
          tunnel: [w271] -> w257
          tunnel: w247 -> [w264]
          stop <- w272 stop-if-true
          w274 = 0.5 ("y")
          # "ask rich about battery power and is it diplayed"
          n168 = local read "EQF1259 com port"() -> (w285:refnum<visa-resource-name>)
          n169 = call "usbUart.vi"("VISA resource name"=w285, "write buffer"="n\u0002", "error in (no error)"=w264) -> ("number[0]"=w299:u32)  [unwired: 1 in, 15 out]
          n170 = call "usbUart.vi"("VISA resource name"=w285, "write buffer"="l\u0002", "error in (no error)"=w264) -> ("number[0]"=w302:u32)  [unwired: 1 in, 15 out]
          n171 = Number To Decimal String(number=w302) -> (decimal integer string=w282:string)  [unwired: 1 in]
          n172 = Number To Decimal String(number=w299) -> (decimal integer string=w297:string)  [unwired: 1 in]
          n173 = String Length(string=w297) -> (length=w295:i32)
          n174 = String Length(string=w282) -> (length=w283:i32)
          n175 = Reverse String(1:w297) -> (0:w291:string)
          n176 = case shown="1, Default" w295 {
            tunnel: ["00" "0" ""] -> w296
            frame 1, Default {
            }
            frame 2 {
            }
            frame 3 {
            }
          }
          n177 = case shown="3" w283 {
            tunnel: w282 -> [w303 w310]
            tunnel: [w305 w312] -> w281
            tunnel: [w304 w311] -> w280
            frame 2, Default {
              n178 = Reverse String(1:w303) -> (0:w308:string)
              n179 = Search/Split String(string=w303, offset (0)=1) -> (substring before match=w305:string)  [unwired: 1 in, 2 out]
              n180 = Search/Split String(string=w308, offset (0)=1) -> (substring before match=w309:string)  [unwired: 1 in, 2 out]
              n181 = Reverse String(1:w309) -> (0:w304:string)
            }
            frame 3 {
              n182 = Reverse String(1:w310) -> (0:w315:string)
              n183 = Search/Split String(string=w310, offset (0)=2) -> (substring before match=w312:string)  [unwired: 1 in, 2 out]
              n184 = Search/Split String(string=w315, offset (0)=1) -> (substring before match=w316:string)  [unwired: 1 in, 2 out]
              n185 = Reverse String(1:w316) -> (0:w311:string)
            }
          }
          n186 = Search/Split String(string=w291, offset (0)=2) -> (substring before match=w292:string)  [unwired: 1 in, 2 out]
          n187 = Reverse String(1:w292) -> (0:w294:string)
          n188 = Concatenate Strings(w296, w297) -> (w298:string)
          n189 = Search/Split String(string=w298, offset (0)=1) -> (substring before match=w293:string)  [unwired: 1 in, 2 out]
          n190 = global read "Global_usbComm.vi" "ConsoleVoltage"() -> (w278:string)
          n191 = Decimal String To Number(string=w278) -> (number=w277:i32)  [unwired: 2 in, 1 out]
          n192 = Concatenate Strings(w293, "." ("string"), w294) -> (w284:string)
          "Current" <- w284
          n193 = Concatenate Strings(w281, "." ("string"), w280) -> (w279:string)
          "Voltage" <- w279
          n194 = To Double Precision Float(number=w277) -> (double precision float=w275:dbl)
          n195 = Add(x=w275, y=w274) -> (x+y=w276:dbl)
          n196 = Subtract(x=w275, y=w274) -> (x-y=w273:dbl)
          n197 = Fract/Exp String To Number(string=w284) -> (number=w266:dbl)  [unwired: 3 in, 1 out]
          n198 = Fract/Exp String To Number(string=w279) -> (number=w267:dbl)  [unwired: 3 in, 1 out]
          n199 = In Range and Coerce(upper limit=w276, x=w267, lower limit=w273) -> (In Range?=→"PowerOn":bool)  [unwired: 1 out]
          n200 = Not Equal To 0?(x=w266) -> (x != 0?=w263:bool)
          "CurrentOn" <- w263
          n201 = Bundle(w267, w266) -> (→"Power On":cluster{dbl, dbl})  [unwired: 1 in]
          n202 = Or(x="Pow1", y="Pow0") -> (x .or. y?=w272:bool)
          n203 = Not(x="Pow0") -> (.not. x?=w269:bool)
          n204 = Compound Arithmetic op=AND(w263, "Pow1", w269) -> (w271:bool)
        }
        n205 = local read "refnum out"() -> (w262:refnum<file>)
        n206 = call "dataSampled.vi"("Data"=w261, "refnum in"=w262) -> ("refnum out"=w259:refnum<file>)  [unwired: 8 in, 1 out]
        n207 = call "dataSampled.vi"("Data"=w260, "refnum in"=w259) -> ()  [unwired: 8 in, 2 out]
        n208 = Select(t=T1."BLEConnect" ("Tab Control"), s=w257, f=T1."Failed" ("Tab Control")) -> (s? t:f=w258:T1)
      }
      frame "BLEConnect" {
        w324 = FALSE
        n209 = local write "BLE0"(w324) -> ()
        n210 = local write "BLE1"(w324) -> ()
        n211 = flat-sequence {
          tunnel: [w334] -> w320
          frame #0 {
            n212 = global read "Global_usbComm.vi" "Display"() -> (w330)
            n213 = Equal?(x=w330, y="0") -> (x = y?=w328:bool)
            n214 = case shown="False" w328 {
              frame False {
                n215 = local read "EQF1259 com port"() -> (w332:refnum<visa-resource-name>)
                n216 = call "usbUart.vi"("VISA resource name"=w332, "write buffer"="S\u0002") -> ()  [unwired: 2 in, 16 out]
              }
              frame True {
                n217 = global write "Global_usbComm.vi" "BLE"("0" ("BLE")) -> ()
              }
            }
          }
          frame #1 {
            n218 = global read "Global_usbComm.vi" "BLE"() -> (w337:string)
            n219 = Equal?(x=w337, y="1") -> (x = y?=w335:bool)
            n220 = while {
              tunnel: [w338] -> w334
              tunnel: w335 -> [w339]
              tunnel: [w338] -> _
              stop <- w341 stop-if-true
              n221 = case shown="True" w339 {
                tunnel: [w342 w344] -> w338
                tunnel: [w342 "BLE1"] -> w340
                frame False {
                  w342 = TRUE
                  n222 = local read "refnum out"() -> (w343:refnum<file>)
                  n223 = call "dataSampled.vi"("refnum in"=w343) -> ()  [unwired: 9 in, 2 out]
                }
                frame True {
                  n224 = global read "Global_usbComm.vi" "PIP_Instruction"() -> (w351:string[][])
                  n225 = Index Array(array=w351, index (row) #1=1 ("index (row)"), index (col) #1=2 ("disabled index (col)"), index (row) #2=1 ("index (row)"), index (col) #2=7 ("disabled index (col)")) -> (element #1=w350:string, element #2=w349:string)
                  "BLE_SETUP-2" <- w350
                  "BLE_CONNECT-7" <- w349
                  n226 = global write "Global_usbComm.vi" "BLE_SETUP-2"(w350) -> ()
                  n227 = global write "Global_usbComm.vi" "BLE_CONNECT-7"(w349) -> ()
                  n228 = Not(x="BLE1") -> (.not. x?=w353:bool)
                  n229 = And(x="BLE0", y=w353) -> (x .and. y?=w344:bool)
                }
              }
              n230 = Or(x=w338, y=w340) -> (x .or. y?=w341:bool)
            }
          }
        }
        n231 = local read "refnum out"() -> (w321:refnum<file>)
        n232 = call "Pass_Fail.vi"("OK"=w320, "Byte Stream File in"=w321) -> ()  [unwired: 8 in, 2 out]
        n233 = Select(t=T1."Maintenance" ("Tab Control"), s=w320, f=T1."Failed" ("Tab Control")) -> (s? t:f=w327:T1)
      }
      frame "Maintenance" {
        w359 = FALSE
        w358 = FALSE
        n234 = local write "Enter Firmware"("") -> ()
        n235 = local write "Cal0"(w358) -> ()
        n236 = local write "Dis0"(w358) -> ()
        n237 = local write "key0"(w358) -> ()
        n238 = local write "Cal1"(w359) -> ()
        n239 = local write "Dis1"(w359) -> ()
        n240 = local write "key1"(w359) -> ()
        n241 = flat-sequence {
          tunnel: [w369] -> w357
          frame #0 {
            n242 = local read "EQF1259 com port"() -> (w365:refnum<visa-resource-name>)
            n243 = call "usbUart.vi"("VISA resource name"=w365, "write buffer"="š\u0001") -> ("PartNumber"=→"decimal integer string":string)  [unwired: 2 in, 15 out]
          }
          frame #1 {
            n244 = local read "EQF1259 com port"() -> (w368:refnum<visa-resource-name>)
            n245 = call "usbUart.vi"("VISA resource name"=w368, "write buffer"="P\u0002") -> ()  [unwired: 2 in, 16 out]
          }
          frame #2 {
            n246 = while {
              shift-right: [w373] -> _
              shift-left: 0 -> [w374]
              tunnel: [w371] -> w369
              stop <- w372 stop-if-true
              n247 = case shown="3" w374 {
                tunnel: [1 2 3 4 5 6 _] -> w373
                tunnel: [FALSE _ _ _ _ _ w426] -> w372
                tunnel: [FALSE _ _ _ _ _ w427] -> w371
                frame 0, Default {
                  n248 = local read "EQF1259 com port"() -> (w377:refnum<visa-resource-name>)
                  n249 = call "usbUart.vi"("VISA resource name"=w377, "write buffer"="@\u0001") -> ("PartNumber"=w376:string)  [unwired: 2 in, 15 out]
                  n250 = call "usbUart.vi"("VISA resource name"=w377, "write buffer"="[\u0004") -> ("BB FW"=w383:string)  [unwired: 2 in, 15 out]
                  n251 = call "usbUart.vi"("VISA resource name"=w377, "write buffer"="\u0001") -> ("PartNumber"=w384:string)  [unwired: 2 in, 15 out]
                  n252 = global write "Global_usbComm.vi" "ButtonType"(w384) -> ()
                  n253 = global write "Global_usbComm.vi" "Firmware"(w383) -> ()
                  n254 = global write "Global_usbComm.vi" "DeviceType"(w376) -> ()
                }
                frame 1 {
                  n255 = local read "decimal integer string"() -> (w386:string)
                  n256 = for {
                    N: 2 -> [_]
                    tunnel: [w393] -> w389
                    n257 = call "maintenancePIP.vi"() -> ("MAINTENANCE MODE-8, 9, 10, 11"=w393:string)  [unwired: 10 in, 1 out]
                  }
                  "MAINTENANCE MODE-8, 9, 10, 11" <- w389
                  n258 = global write "Global_usbComm.vi" "TABLET"(w386) -> ()
                  n259 = global read "Global_usbComm.vi" "GRADE"() -> (w385:string)
                  n260 = case shown="\"1\", Default" w385 {
                    frame "1", Default {
                      w390 = TRUE
                      n261 = property on="Cal1" class="Bool (strict)"("Visible"=w390) -> ()  [unwired: 2 in, 2 out]
                      n262 = property on="Cal0" class="Bool (strict)"("Visible"=w390) -> ()  [unwired: 2 in, 2 out]
                    }
                    frame "0" {
                      w391 = FALSE
                      n263 = local write "Cal1"(TRUE) -> ()
                      n264 = property on="Cal1" class="Bool (strict)"("Visible"=w391) -> ()  [unwired: 2 in, 2 out]
                      n265 = property on="Cal0" class="Bool (strict)"("Visible"=w391) -> ()  [unwired: 2 in, 2 out]
                    }
                  }
                }
                frame 2 {
                  n266 = while {
                    tunnel: ["Enter Firmware"] -> w394
                    stop <- w399 stop-if-true
                    n267 = control-ref of="Enter Firmware"() -> (w398:refnum<vi>)
                    n268 = call "focusKey_input.vi"("reference"=w398) -> ()  [unwired: 10 in, 1 out]
                    n269 = Empty String/Path?(string/path="Enter Firmware") -> (empty?=w400:bool)
                    n270 = Not(x=w400) -> (.not. x?=w399:bool)
                  }
                  n271 = local read "refnum out"() -> (w395:refnum<file>)
                  n272 = call "dataSampled.vi"("Data"=w394, "refnum in"=w395) -> ()  [unwired: 8 in, 2 out]
                }
                frame 3 {
                  n273 = local read "EQF1259 com port"() -> (w402:refnum<visa-resource-name>)
                  n274 = call "Elapsed Time5"() -> ("Time has Elapsed"=w401:bool)  [unwired: 12 in, 7 out]
                  n275 = call "inclineCalibrate.vi"("VISA Refnum in"=w402) -> ("Complete"=w403:bool)  [unwired: 8 in, 2 out]
                  n276 = local write "Cal1"(w403) -> ()
                  n277 = local write "Cal0"(w401) -> ()
                  n278 = Not(x="Cal0") -> (.not. x?=w406:bool)
                  n279 = And(x="Cal1", y=w406) -> (x .and. y?=w409:bool)
                  n280 = local read "refnum out"() -> (w408:refnum<file>)
                  n281 = call "Pass_Fail.vi"("OK"=w409, "Byte Stream File in"=w408) -> ()  [unwired: 8 in, 2 out]
                }
                frame 4 {
                  n282 = while {
                    tunnel: [w416] -> w412
                    stop <- w415 stop-if-true
                    n283 = Or(x="Dis1", y="Dis0") -> (x .or. y?=w415:bool)
                    n284 = Not(x="Dis0") -> (.not. x?=w417:bool)
                    n285 = And(x="Dis1", y=w417) -> (x .and. y?=w416:bool)
                  }
                  n286 = local read "refnum out"() -> (w411:refnum<file>)
                  n287 = call "Pass_Fail.vi"("OK"=w412, "Byte Stream File in"=w411) -> ()  [unwired: 8 in, 2 out]
                }
                frame 5 {
                  n288 = while {
                    tunnel: [w424] -> w419
                    stop <- w423 stop-if-true
                    n289 = Or(x="key1", y="key0") -> (x .or. y?=w423:bool)
                    n290 = Not(x="key0") -> (.not. x?=w425:bool)
                    n291 = And(x="key1", y=w425) -> (x .and. y?=w424:bool)
                  }
                  n292 = local read "refnum out"() -> (w418:refnum<file>)
                  n293 = call "Pass_Fail.vi"("OK"=w419, "Byte Stream File in"=w418) -> ()  [unwired: 8 in, 2 out]
                }
                frame 6 {
                  n294 = while {
                    tunnel: [w429] -> w427
                    tunnel: [w428] -> w426
                    stop <- w428 stop-if-true
                    n295 = local read "key1"() -> (w433:bool)
                    n296 = local read "Cal1"() -> (w431:bool)
                    n297 = local read "Dis1"() -> (w432:bool)
                    n298 = Compound Arithmetic op=OR(w431, w432, w433) -> (w429:bool)
                    n299 = Not(x=w429) -> (.not. x?=w430:bool)
                    n300 = Or(x=w429, y=w430) -> (x .or. y?=w428:bool)
                  }
                }
              }
            }
          }
        }
        n301 = Select(t=T1."PWM/Tach" ("Tab Control"), s=w357, f=T1."Failed" ("Tab Control")) -> (s? t:f=w363:T1)
      }
      frame "PWM/Tach" {
        w442 = FALSE ("stop")
        w441 = 0.0 ("SPEED")
        w443 = ""
        n302 = local write "SPEED TREADMILL"(w441) -> ()
        n303 = local write "MaxSpeed Time (s)"(w441) -> ()
        n304 = local write "E-Stop"(w442) -> ()
        n305 = local write "Smin"(w442) -> ()
        n306 = local write "Smid"(w442) -> ()
        n307 = local write "Smax"(w442) -> ()
        n308 = local write "PWM"(w443) -> ()
        n309 = local write "MID"(w443) -> ()
        n310 = local write "START"(w443) -> ()
        n311 = local read "EQF1259 com port"() -> (w437:refnum<visa-resource-name>)
        n312 = local write "FREQUENCY"(w443) -> ()
        n313 = call "usbUart.vi"("VISA resource name"=w437, "write buffer"="@\u0001") -> ("number[0]"=w436:u32)  [unwired: 2 in, 15 out]
        n314 = case shown="1" w436 {
          tunnel: [w455 w513] -> w445
          tunnel: [w454 w510] -> w444
          frame 1 {
            w457 = TRUE
            w456 = FALSE ("Visible")
            n315 = property on="Tac1" class="Bool (strict)"("Visible"=w457) -> ()  [unwired: 2 in, 2 out]
            n316 = property on="Tac0" class="Bool (strict)"("Visible"=w457) -> ()  [unwired: 2 in, 2 out]
            n317 = property on="Smin" class="Bool (strict)"("Visible"=w456) -> ()  [unwired: 2 in, 2 out]
            n318 = property on="START" class="Str"("Visible"=w456) -> ()  [unwired: 2 in, 2 out]
            n319 = property on="MPH/KPH" class="Str"("Visible"=w456) -> ()  [unwired: 2 in, 2 out]
            n320 = property on="Smid" class="Bool (strict)"("Visible"=w456) -> ()  [unwired: 2 in, 2 out]
            n321 = property on="MID" class="Str"("Visible"=w456) -> ()  [unwired: 2 in, 2 out]
            n322 = property on="Smax" class="Bool (strict)"("Visible"=w456) -> ()  [unwired: 2 in, 2 out]
            n323 = property on="MAX" class="Str"("Visible"=w456) -> ()  [unwired: 2 in, 2 out]
            n324 = property on="PWM" class="Str"("Visible"=w456) -> ()  [unwired: 2 in, 2 out]
            n325 = local write "Tac0"(w456) -> ()
            n326 = local write "Tac1"(w456) -> ()
            n327 = property on="RPM AEROBIC" class="Knob (strict)"("Visible"=w457) -> ()  [unwired: 2 in, 2 out]
            n328 = property on="SPEED AEROBIC" class="Knob (strict)"("Visible"=w457) -> ()  [unwired: 2 in, 2 out]
            n329 = property on="SPEED TREADMILL" class="Knob (strict)"("Visible"=w456) -> ()  [unwired: 2 in, 2 out]
            n330 = property on="FREQUENCY" class="Str"("Visible"=w456) -> ()  [unwired: 2 in, 2 out]
            n331 = flat-sequence {
              tunnel: [w466] -> w453
              tunnel: [w464] -> w450
              tunnel: w453 -> [w475]
              tunnel: w450 -> [w474]
              tunnel: [w474] -> w449
              tunnel: [w473] -> w448
              tunnel: [w472] -> w447
              tunnel: w449 -> [w478]
              frame #0 {
                n332 = local read "EQF1259 com port"() -> (w464:refnum<visa-resource-name>)
                n333 = call "usbUart.vi"("VISA resource name"=w464, "write buffer"="›\u0001") -> ("PartNumber"=w467:string, "error out"=w465:errorcluster)  [unwired: 2 in, 14 out]
                n334 = global write "Global_usbComm.vi" "distanceType"(w467) -> ()
                n335 = call "usbUart.vi"("VISA resource name"=w464, "write buffer"="@\u0001", "error in (no error)"=w465) -> ("PartNumber"=w468:string, "error out"=w466:errorcluster)  [unwired: 1 in, 14 out]
                n336 = global write "Global_usbComm.vi" "DeviceType"(w468) -> ()
              }
              frame #1 {
                n337 = call "pwm_rpmPIP.vi"("error in (no error)"=w475) -> ("error out"=w471:errorcluster, "PWM_RPM"=w476:string)  [unwired: 9 in]
                n338 = local write "PWM_RPM"(w476) -> ()
                n339 = call "Display Message to User5"("error in (no error)"=w471) -> ("error out"=w473:errorcluster, "OK"=w472:bool)  [unwired: 9 in]
              }
              frame #2 {
                n340 = call "usbUart.vi"("VISA resource name"=w478, "write buffer"="\u0005\u0004") -> ()  [unwired: 2 in, 16 out]
              }
            }
            n341 = while {
              tunnel: w447 -> [w488]
              tunnel: [w487] -> w451
              tunnel: [w486] -> w452
              tunnel: [w483] -> w455
              tunnel: [w482] -> w454
              tunnel: w448 -> [w481]
              stop <- w485 stop-if-true
              n342 = feedback #1() -> (w484:bool)  [unwired: 1 in]
              n343 = case shown="True" w488 {
                tunnel: [w490 w499] -> w485
                tunnel: [w491 w503] -> w487
                tunnel: [w491 w502] -> w486
                tunnel: w484 -> [_ w501]
                tunnel: [w490 w494] -> w483
                tunnel: [FALSE ("E-Stop") w493] -> w482
                tunnel: w481 -> [_ w492]
                frame False {
                  w491 = ""
                  w490 = TRUE
                }
                frame True {
                  n344 = call "Elapsed Time"("Reset"=w501) -> ("Elapsed Time (s)"=w504:dbl, "Time has Elapsed"=w500:bool)  [unwired: 11 in, 6 out]
                  n345 = local write "MaxSpeed Time (s)"(w504) -> ()
                  n346 = local read "EQF1259 com port"() -> (w507:refnum<visa-resource-name>)
                  n347 = call "speedSet.vi"("error in (no error)"=w492, "VISA resource name"=w507) -> (2:"RPM"=w502:string, "Speed"=w503:string, 4:"RPM"=→"RPM AEROBIC":dbl, "SPEED"=→"SPEED AEROBIC":dbl)  [unwired: 5 in, 1 out]
                  n348 = local read "E-Stop"() -> (w493:bool)
                  n349 = Or(x="Tac1", y="Tac0") -> (x .or. y?=w495:bool)
                  n350 = Not(x="Tac0") -> (.not. x?=w498:bool)
                  n351 = And(x="Tac1", y=w498) -> (x .and. y?=w494:bool)
                  n352 = Compound Arithmetic op=OR(w495, w493, w500) -> (w499:bool)
                }
              }
              n353 = feedback-in #1(w485) -> ()
            }
            n354 = local read "refnum out"() -> (w462:refnum<file>)
            n355 = call "dataSampled.vi"("Data"=w451, "refnum in"=w462) -> ("error out"=w459:errorcluster, "refnum out"=w463:refnum<file>)  [unwired: 8 in]
            n356 = call "dataSampled.vi"("Error In"=w459, "Data"=w452, "refnum in"=w463) -> ("error out"=w460:errorcluster, "refnum out"=w461:refnum<file>)  [unwired: 7 in]
            n357 = for {
              N: 5 -> [_]
              tunnel: w461 -> [w480]
              tunnel: w460 -> [w479]
              n358 = call "dataSampled.vi"("Error In"=w479, "refnum in"=w480) -> ()  [unwired: 8 in, 2 out]
            }
          }
          frame 0, Default {
            w508 = FALSE
            w509 = TRUE ("Visible")
            n359 = property on="Tac1" class="Bool (strict)"("Visible"=w508) -> ()  [unwired: 2 in, 2 out]
            n360 = property on="Tac0" class="Bool (strict)"("Visible"=w508) -> ()  [unwired: 2 in, 2 out]
            n361 = for {
              N: 2 -> [_]
              tunnel: [w520] -> w517
              tunnel: [w519] -> w511
              n362 = flat-sequence {
                tunnel: [w555] -> w520
                tunnel: [w549] -> w519
                frame #0 {
                  n363 = local read "EQF1259 com port"() -> (w525:refnum<visa-resource-name>)
                  n364 = local read "EQF1259 com port"() -> (w527:refnum<visa-resource-name>)
                  n365 = call "usbUart.vi"("VISA resource name"=w525, "write buffer"="v\u0002") -> ("maxSpeed"=w521:string)  [unwired: 2 in, 15 out]
                  n366 = call "usbUart.vi"("VISA resource name"=w527, "write buffer"="E\u0001") -> ("PartNumber"=w523:string)  [unwired: 2 in, 15 out]
                  n367 = Fract/Exp String To Number(string=w521) -> (number=w522:dbl)  [unwired: 3 in, 1 out]
                  n368 = global write "Global_usbComm.vi" "UnitType"(w523) -> ()
                  n369 = case shown="\"1\", Default" w523 {
                    tunnel: w522 -> [w536 w544]
                    tunnel: w521 -> [_ w538]
                    frame "1", Default {
                      # "euro"
                      n370 = local write "lower"(2.0) -> ()
                      n371 = local write "upper"(2.3) -> ()
                      n372 = local write "middle"(0.5) -> ()
                      n373 = Multiply(x=w536, y=1.60934) -> (x*y=w533:dbl)
                      n374 = Number To Fractional String(number=w533, precision (6)=i16 1) -> (F-format string=w534:string)  [unwired: 2 in]
                      "MAX" <- w534
                      n375 = Subtract(x=w533, y=0.6) -> (x-y=w531:dbl)
                      n376 = local write "minMax"(w531) -> ()
                      n377 = global write "Global_usbComm.vi" "MaxSpeed"(w534) -> ()
                    }
                    frame "2" {
                      # "dom"
                      n378 = local write "MAX"(w538) -> ()
                      n379 = global write "Global_usbComm.vi" "MaxSpeed"(w538) -> ()
                      n380 = Subtract(x=w544, y=0.5) -> (x-y=→"minMax":dbl)
                      "lower" <- 1.0
                      "middle" <- 0.5
                      "upper" <- 1.2
                    }
                  }
                }
                frame #1 {
                  w545 = 0.2 ("y")
                  # "mid limit"
                  n381 = global read "Global_usbComm.vi" "MaxSpeed"() -> (w551:string)
                  n382 = Fract/Exp String To Number(string=w551) -> (number=w553:dbl)  [unwired: 3 in, 1 out]
                  "MAX" <- w553
                  n383 = Divide(x=w553, y=2.0) -> (x/y=w546:dbl)
                  n384 = Add(x=w553, y=2.0) -> (x+y=w549:dbl)
                  n385 = Subtract(x=w546, y=w545) -> (x-y=→"lowerLimit":dbl)
                  n386 = Add(x=w546, y=w545) -> (x+y=→"upperLimit":dbl)
                  n387 = call "pwm_rpmPIP.vi"() -> ("error out"=w555:errorcluster, "PWM_RPM"=→"PWM_RPM":string)  [unwired: 10 in]
                }
              }
            }
            n388 = property on="Smin" class="Bool (strict)"("Visible"=w509) -> ()  [unwired: 2 in, 2 out]
            n389 = property on="START" class="Str"("Visible"=w509) -> ()  [unwired: 2 in, 2 out]
            n390 = property on="MPH/KPH" class="Str"("Visible"=w509) -> ()  [unwired: 2 in, 2 out]
            n391 = property on="Smid" class="Bool (strict)"("Visible"=w509) -> ()  [unwired: 2 in, 2 out]
            n392 = property on="MID" class="Str"("Visible"=w509) -> ()  [unwired: 2 in, 2 out]
            n393 = property on="Smax" class="Bool (strict)"("Visible"=w509) -> ()  [unwired: 2 in, 2 out]
            n394 = property on="MAX" class="Str"("Visible"=w509) -> ()  [unwired: 2 in, 2 out]
            n395 = property on="PWM" class="Str"("Visible"=w509) -> ()  [unwired: 2 in, 2 out]
            n396 = property on="RPM AEROBIC" class="Knob (strict)"("Visible"=w508) -> ()  [unwired: 2 in, 2 out]
            n397 = property on="SPEED AEROBIC" class="Knob (strict)"("Visible"=w508) -> ()  [unwired: 2 in, 2 out]
            n398 = property on="SPEED TREADMILL" class="Knob (strict)"("Visible"=w509) -> ()  [unwired: 2 in, 2 out]
            n399 = property on="FREQUENCY" class="Str"("Visible"=w509) -> ()  [unwired: 2 in, 2 out]
            n400 = property on="SPEED TREADMILL" class="Knob (strict)"(error in=w517, "Scale.Maximum"=w511) -> (error out=w518:errorcluster)  [unwired: 1 in, 1 out]
            n401 = local read "EQF1259 com port"() -> (w515:refnum<visa-resource-name>)
            n402 = call "Display Message to User"("error in (no error)"=w518) -> ("error out"=w512:errorcluster)  [unwired: 9 in, 1 out]
            n403 = local read "refnum out"() -> (w516:refnum<file>)
            n404 = while {
              tunnel: w516 -> [w579]
              tunnel: w515 -> [w565]
              tunnel: w512 -> [w576]
              tunnel: [w572] -> w513
              tunnel: ["E-Stop"] -> w510
              stop <- w563 stop-if-true
              n405 = call "speedAquire.vi"("error in (no error)"=w576, "VISA resource name"=w565) -> ("error out (no error)"=w578:errorcluster, "FREQUENCY"=w575:string, "PWM"=w577:string, "KPH/MPH"=→"MPH/KPH":string, "SPEED"=w556:dbl)  [unwired: 5 in]
              "SPEED TREADMILL" <- w556
              "FREQUENCY" <- w575
              "PWM" <- w577
              n406 = local read "upperLimit"() -> (w557:dbl)
              n407 = local read "lowerLimit"() -> (w558:dbl)
              n408 = local read "upper"() -> (w559:dbl)
              n409 = local read "lower"() -> (w560:dbl)
              n410 = In Range and Coerce(upper limit=w557, x=w556, lower limit=w558) -> (In Range?=w573:bool)  [unwired: 1 out]
              n411 = In Range and Coerce(upper limit=w559, x=w556, lower limit=w560) -> (In Range?=w574:bool)  [unwired: 1 out]
              n412 = case shown="True" w574 {
                tunnel: [w620 w627] -> w583
                tunnel: [w621 w629] -> w581
                tunnel: w579 -> [w621 w632]
                tunnel: w578 -> [w620 _]
                tunnel: w577 -> [_ w628]
                tunnel: w556 -> [_ w624]
                frame False {
                }
                frame True {
                  n413 = Number To Fractional String(number=w624, precision (6)=i16 1) -> (F-format string=w623:string)  [unwired: 2 in]
                  "START" <- w623
                  n414 = Wait (ms)(milliseconds to wait=u32 1500) -> ()  [unwired: 1 out]
                  n415 = call "dataSampled.vi"("Data"=w623, "refnum in"=w632) -> ("error out"=w631:errorcluster, "refnum out"=w630:refnum<file>)  [unwired: 8 in]
                  n416 = call "dataSampled.vi"("Error In"=w631, "Data"=w628, "refnum in"=w630) -> ("error out"=w627:errorcluster, "refnum out"=w629:refnum<file>)  [unwired: 7 in]
                  "Smin" <- TRUE
                }
              }
              n417 = case shown="True" w573 {
                tunnel: [w606 w614] -> w582
                tunnel: w583 -> [w606 w619]
                tunnel: w581 -> [w607 w618]
                tunnel: [w607 w615] -> w580
                tunnel: w577 -> [_ w613]
                tunnel: w556 -> [_ w609]
                frame False {
                }
                frame True {
                  n418 = Number To Fractional String(number=w609, precision (6)=i16 1) -> (F-format string=w610:string)  [unwired: 2 in]
                  "MID" <- w610
                  n419 = Wait (ms)(milliseconds to wait=u32 1500) -> ()  [unwired: 1 out]
                  n420 = call "dataSampled.vi"("Error In"=w619, "Data"=w610, "refnum in"=w618) -> ("error out"=w617:errorcluster, "refnum out"=w616:refnum<file>)  [unwired: 7 in]
                  n421 = call "dataSampled.vi"("Error In"=w617, "Data"=w613, "refnum in"=w616) -> ("error out"=w614:errorcluster, "refnum out"=w615:refnum<file>)  [unwired: 7 in]
                  "Smid" <- TRUE
                }
              }
              n422 = local read "minMax"() -> (w561:dbl)
              n423 = local read "MAX"() -> (w562:dbl)
              n424 = In Range and Coerce(upper limit=w562, x=w556, lower limit=w561) -> (In Range?=w569:bool)  [unwired: 1 out]
              n425 = case shown="True" w569 {
                tunnel: w582 -> [w592 w605]
                tunnel: w580 -> [_ w604]
                tunnel: w577 -> [_ w601]
                tunnel: w575 -> [_ w598]
                tunnel: [w592 w596] -> w571
                tunnel: w556 -> [_ w594]
                frame False {
                }
                frame True {
                  n426 = Number To Fractional String(number=w594, precision (6)=i16 1) -> (F-format string=w595:string)  [unwired: 2 in]
                  n427 = call "dataSampled.vi"("Error In"=w605, "Data"=w595, "refnum in"=w604) -> ("error out"=w603:errorcluster, "refnum out"=w602:refnum<file>)  [unwired: 7 in]
                  n428 = call "dataSampled.vi"("Error In"=w603, "Data"=w601, "refnum in"=w602) -> ("error out"=w600:errorcluster, "refnum out"=w599:refnum<file>)  [unwired: 7 in]
                  n429 = call "dataSampled.vi"("Error In"=w600, "Data"=w598, "refnum in"=w599) -> ("error out"=w596:errorcluster)  [unwired: 7 in, 1 out]
                  "Smax" <- TRUE
                }
              }
              n430 = feedback #2() -> (w564:bool)  [unwired: 1 in]
              n431 = call "Elapsed Time2"("Reset"=w564) -> ("Elapsed Time (s)"=→"MaxSpeed Time (s)":dbl, "Time has Elapsed"=w568:bool)  [unwired: 11 in, 6 out]
              n432 = Compound Arithmetic op=OR("E-Stop", w569, w568) -> (w563:bool)
              n433 = feedback-in #2(w563) -> ()
              n434 = while {
                tunnel: [w585] -> w572
                tunnel: w571 -> [w584]
                stop <- w587 stop-if-true
                n435 = call <vilib>:"Simple Error Handler.vi"("error in (no error)"=w584) -> ()  [unwired: 4 in, 5 out]
                n436 = local read "Smax"() -> (w588:bool)
                n437 = local read "Smin"() -> (w590:bool)
                n438 = local read "Smid"() -> (w589:bool)
                n439 = Compound Arithmetic op=AND(TRUE ("value"), w590, w589, w588) -> (w585:bool)
                n440 = Not(x=w585) -> (.not. x?=w586:bool)
                n441 = Or(x=w586, y=w585) -> (x .or. y?=w587:bool)
              }
            }
          }
        }
        n442 = Select(t=T1."Pulse" ("Tab Control"), s=w445, f=T1."Failed" ("Tab Control")) -> (s? t:f=w446:T1)
      }
      frame "Incline" {
        n443 = local write "negative incline"(0.0 ("negative incline")) -> ()
        n444 = for {
          N: 2 -> [_]
          tunnel: [w652] -> w635
          tunnel: [w646] -> w636
          w650 = 0.1 ("y")
          w651 = FALSE
          # "percent\nmax incline\nmin incline"
          n445 = local write "INCLINE"(0.0 ("INCLINE")) -> ()
          n446 = local read "EQF1259 com port"() -> (w654:refnum<visa-resource-name>)
          n447 = property on="INCLINE" class="WFChart (strict)"("History Data"=dbl[] []) -> ()  [unwired: 2 in, 2 out]
          n448 = local write "Imax"(w651) -> ()
          n449 = local write "Imin"(w651) -> ()
          n450 = local write "Imid"(w651) -> ()
          n451 = local write "E-Stop/Incline"(w651) -> ()
          n452 = local write "resultIncline"(w651) -> ()
          n453 = call "usbUart.vi"("VISA resource name"=w654, "write buffer"="€\u0002") -> ("number[0]"=w661:u32, "error out"=w653:errorcluster)  [unwired: 2 in, 14 out]
          n454 = call "usbUart.vi"("VISA resource name"=w654, "write buffer"="‚\u0002", "error in (no error)"=w653) -> ("number[0]"=w657:u32, "negative incline"=w656:dbl, "error out"=w652:errorcluster)  [unwired: 1 in, 13 out]
          n455 = Equal?(x=w657, y=u32 0) -> (x = y?=w658:bool)
          n456 = case shown="False" w658 {
            tunnel: w657 -> [_ w672]
            tunnel: w656 -> [w670 _]
            tunnel: [w670 w671] -> w655
            frame False {
              "negative incline" <- w670
            }
            frame True {
              n457 = To Double Precision Float(number=w672) -> (double precision float=w671:dbl)
            }
          }
          n458 = To Double Precision Float(number=w661) -> (double precision float=w666:dbl)
          n459 = Multiply(x=w666, y=w650) -> (x*y=w665:dbl)
          "inclineMax" <- w665
          n460 = Multiply(x=w655, y=w650) -> (x*y=w649:dbl)
          "inclineMin" <- w649
          n461 = global read "Global_usbComm.vi" "Controller/PowerBoard"() -> (w648:string)
          n462 = Add(x=w665, y=w649) -> (x+y=w664:dbl)
          n463 = Divide(x=w664, y=2.0) -> (x/y=→"inclineMid":dbl)
          n464 = Not Equal?(x=w648, y="0") -> (x != y?=w646:bool)
        }
        n465 = call "inclinePIP.vi"("error in (no error)"=w635, "Boolean"=w636) -> ("error out"=w634:errorcluster, "String"=→"INCLINE-14":string)  [unwired: 8 in]
        n466 = case shown="True" w636 {
          tunnel: [TRUE w679] -> w644
          tunnel: [FALSE ("E-Stop/Incline") w678] -> w643
          tunnel: w634 -> [_ w682]
          frame False {
            n467 = local read "refnum out"() -> (w676:refnum<file>)
            n468 = call "dataSampled.vi"("refnum in"=w676) -> ("refnum out"=w675:refnum<file>)  [unwired: 9 in, 1 out]
            n469 = call "dataSampled.vi"("refnum in"=w675) -> ("refnum out"=w674:refnum<file>)  [unwired: 9 in, 1 out]
            n470 = call "dataSampled.vi"("refnum in"=w674) -> ()  [unwired: 9 in, 2 out]
          }
          frame True {
            n471 = call "Display Message to User2"("error in (no error)"=w682) -> ("error out"=w683:errorcluster)  [unwired: 9 in, 1 out]
            n472 = while {
              tunnel: ["E-Stop/Incline"] -> w680
              tunnel: [w709] -> w681
              tunnel: w683 -> [w704]
              stop <- w707 stop-if-true
              n473 = local read "EQF1259 com port"() -> (w725:refnum<visa-resource-name>)
              n474 = local read "negative incline"() -> (w702:dbl)
              n475 = call "usbUart.vi"("VISA resource name"=w725, "write buffer"="}\u0002" ("write buffer 2"), "error in (no error)"=w704) -> ("number[0]"=w720:u32, "negative incline"=w719:dbl)  [unwired: 1 in, 14 out]
              n476 = To Double Precision Float(number=w720) -> (double precision float=w722:dbl)
              n477 = Less Or Equal?(x=w719, y=w702) -> (x <= y?=w723:bool)
              n478 = case shown="True" w723 {
                tunnel: w719 -> [w732 _]
                tunnel: w722 -> [_ w733]
                tunnel: [w732 w733] -> w721
                frame False {
                }
                frame True {
                }
              }
              n479 = feedback #3() -> (w708:bool)  [unwired: 1 in]
              n480 = call "Elapsed Time3"("Reset"=w708, "error in (no error)"=w704) -> ("Elapsed Time (s)"=w701:dbl, "Time has Elapsed"=w718:bool)  [unwired: 10 in, 6 out]
              "Incline Time (s)" <- w701
              n481 = global write "Global_usbComm.vi" "tempNumeric"(w701) -> ()
              n482 = local read "inclineMin"() -> (w703:dbl)
              n483 = local read "inclineMid"() -> (w705:dbl)
              n484 = Multiply(x=w721, y=0.1) -> (x*y=w711:dbl)
              "INCLINE" <- w711
              n485 = local read "inclineMax"() -> (w724:dbl)
              n486 = Add(x=0.6, y=w703) -> (x+y=w713:dbl)
              n487 = Add(x=w703, y=0.3) -> (x+y=w710:dbl)
              n488 = Subtract(x=w705, y=0.5) -> (x-y=w706:dbl)
              n489 = local read "refnum out"() -> (w726:refnum<file>)
              n490 = In Range and Coerce(upper limit=w705, x=w711, lower limit=w706) -> (In Range?=w727:bool)  [unwired: 1 out]
              n491 = In Range and Coerce(upper limit=w713, x=w711, lower limit=w710) -> (In Range?=w730:bool)  [unwired: 1 out]
              n492 = Equal?(x=w711, y=w724) -> (x = y?=w709:bool)
              "resultIncline" <- w709
              n493 = case shown="True" w730 {
                tunnel: w711 -> [_ w753]
                tunnel: [w747 w752] -> w729
                tunnel: w726 -> [w747 w751]
                frame False {
                }
                frame True {
                  n494 = Number To Fractional String(number=w753, precision (6)=i16 1) -> (F-format string=w754:string)  [unwired: 2 in]
                  n495 = Wait (ms)(milliseconds to wait=u32 2000) -> ()  [unwired: 1 out]
                  n496 = call "dataSampled.vi"("Data"=w754, "refnum in"=w751) -> ("refnum out"=w752:refnum<file>)  [unwired: 8 in, 1 out]
                  "Imin" <- TRUE
                }
              }
              n497 = Compound Arithmetic op=OR(w709, "E-Stop/Incline", w718) -> (w707:bool)
              n498 = feedback-in #3(w707) -> ()
              n499 = case shown="True" w727 {
                tunnel: w729 -> [w739 w746]
                tunnel: w711 -> [_ w744]
                tunnel: [w739 w743] -> w728
                frame False {
                }
                frame True {
                  n500 = Number To Fractional String(number=w744, precision (6)=i16 1) -> (F-format string=w745:string)  [unwired: 2 in]
                  n501 = Wait (ms)(milliseconds to wait=u32 2000) -> ()  [unwired: 1 out]
                  n502 = call "dataSampled.vi"("Data"=w745, "refnum in"=w746) -> ("refnum out"=w743:refnum<file>)  [unwired: 8 in, 1 out]
                  "Imid" <- TRUE
                }
              }
              n503 = case shown="True" w709 {
                tunnel: w728 -> [_ w738]
                tunnel: w711 -> [_ w736]
                frame False {
                }
                frame True {
                  n504 = Number To Fractional String(number=w736, precision (6)=i16 1) -> (F-format string=w737:string)  [unwired: 2 in]
                  n505 = call "dataSampled.vi"("Data"=w737, "refnum in"=w738) -> ()  [unwired: 8 in, 2 out]
                  "Imax" <- TRUE
                }
              }
            }
            n506 = while {
              tunnel: w681 -> [w699]
              tunnel: w680 -> [w700]
              tunnel: [w699] -> w679
              tunnel: [w700] -> w678
              stop <- w685 stop-if-true
              n507 = global read "Global_usbComm.vi" "tempNumeric"() -> (w691:dbl)
              n508 = feedback #4() -> (w684:bool)  [unwired: 1 in]
              n509 = call "Elapsed Time4"("Reset"=w684) -> ("Elapsed Time (s)"=w694:dbl)  [unwired: 11 in, 7 out]
              n510 = local read "EQF1259 com port"() -> (w697:refnum<visa-resource-name>)
              n511 = Subtract(x=w691, y=w694) -> (x-y=w688:dbl)
              n512 = local write "Incline Time (s)"(w688) -> ()
              n513 = In Range and Coerce(upper limit=0.5, x=w688, lower limit=0.25 ("y")) -> (In Range?=w692:bool)  [unwired: 1 out]
              n514 = call "usbUart.vi"("VISA resource name"=w697, "write buffer"="}\u0002" ("write buffer 2")) -> ("number[0]"=w696:u32)  [unwired: 2 in, 15 out]
              n515 = To Double Precision Float(number=w696) -> (double precision float=w689:dbl)
              n516 = local write "INCLINE"(w689) -> ()
              n517 = In Range and Coerce(upper limit=6.0 ("x"), x=w689, lower limit=4.0) -> (In Range?=w693:bool)  [unwired: 1 out]
              n518 = Or(x=w692, y=w693) -> (x .or. y?=w685:bool)
              n519 = feedback-in #4(w685) -> ()
            }
          }
        }
        n520 = Select(t=T1."CSafe" ("Tab Control"), s=w644, f=T1."Failed" ("Tab Control")) -> (s? t:f=w645:T1)
      }
      frame "Resistance" {
        w758 = FALSE ("overCurrent")
        n521 = local write "current#"("") -> ()
        n522 = property on="RESISTANCE/CURRENT" class="WFChart (strict)"("History Data"=cluster{"number[0]":u32, dbl}[] []) -> ()  [unwired: 2 in, 2 out]
        n523 = local write "RES0"(w758) -> ()
        n524 = local write "RES1"(w758) -> ()
        n525 = local write "RESISTANCE/CURRENT"(cluster{"number[0]":u32, dbl} {"number[0]"=0, 0.0} ("RESISTANCE/CURRENT")) -> ()
        n526 = local write "resistance result"(w758) -> ()
        n527 = local write "ADC low"(w758) -> ()
        n528 = local write "ADC hi"(w758) -> ()
        n529 = local write "ADC mid"(w758) -> ()
        n530 = local write "overCurrent"(w758) -> ()
        n531 = flat-sequence {
          tunnel: [w776] -> w757
          frame #0 {
            n532 = local read "EQF1259 com port"() -> (w766:refnum<visa-resource-name>)
            n533 = call "usbUart.vi"("VISA resource name"=w766, "write buffer"="S\u0002") -> ()  [unwired: 2 in, 16 out]
          }
          frame #1 {
            n534 = global read "Global_usbComm.vi" "RESISTANCE"() -> (w775:string)
            n535 = global read "Global_usbComm.vi" "TABLET"() -> (w773:string)
            n536 = Equal?(x=w775, y="1") -> (x = y?=w771:bool)
            n537 = Not Equal?(x=w773, y="0") -> (x != y?=w770:bool)
            n538 = Compound Arithmetic op=AND(TRUE ("value"), w771, w770) -> (w769:bool)
            n539 = case shown="True" w769 {
              tunnel: [w777 TRUE] -> w776
              frame False {
                n540 = global read "Global_usbComm.vi" "RESISTANCE"() -> (w779:string)
                n541 = Equal?(x=w779, y="1") -> (x = y?=w778:bool)
                n542 = case shown="False" w778 {
                  tunnel: [FALSE TRUE] -> w777
                  frame False {
                  }
                  frame True {
                    n543 = local read "EQF1259 com port"() -> (w784:refnum<visa-resource-name>)
                    n544 = call "usbUart.vi"("VISA resource name"=w784, "write buffer"="\u0005\u0004") -> ()  [unwired: 2 in, 16 out]
                  }
                }
              }
              frame True {
              }
            }
          }
        }
        n545 = while {
          tunnel: w757 -> [w788]
          tunnel: [w786] -> w762
          stop <- w787 stop-if-true
          n546 = case shown="True" w788 {
            tunnel: [w789 w839] -> w787
            tunnel: [w789 w793] -> w786
            frame False {
              w789 = TRUE
              n547 = local read "refnum out"() -> (w792:refnum<file>)
              n548 = call "dataSampled.vi"("refnum in"=w792) -> ("refnum out"=w791:refnum<file>)  [unwired: 9 in, 1 out]
              n549 = call "dataSampled.vi"("refnum in"=w791) -> ("refnum out"=w790:refnum<file>)  [unwired: 9 in, 1 out]
              n550 = call "dataSampled.vi"("refnum in"=w790) -> ()  [unwired: 9 in, 2 out]
            }
            frame True {
              w811 = 120.0
              w810 = 100.0
              w809 = 40.0
              n551 = local read "EQF1259 com port"() -> (w816:refnum<visa-resource-name>)
              n552 = call "usbUart.vi"("VISA resource name"=w816, "write buffer"="‘\u0001" ("write buffer buffer")) -> ("PartNumber"=w812:string, "error out"=w813:errorcluster)  [unwired: 2 in, 14 out]
              n553 = call "usbUart.vi"("VISA resource name"=w816, "write buffer"="n\u0002") -> ("number[0]"=w834:u32)  [unwired: 2 in, 15 out]
              n554 = call "resistancePIP.vi"("Boolean"=TRUE) -> ("error out"=w842:errorcluster, "RESISTANCE-15"=→"RESISTANCE-15":string)  [unwired: 9 in]
              n555 = call "usbUart.vi"("VISA resource name"=w816, "write buffer"="p\u0001", "error in (no error)"=w842) -> ("number[1]"=w854:u32)  [unwired: 1 in, 15 out]
              n556 = Fract/Exp String To Number(string=w812) -> (number=w805:dbl)  [unwired: 3 in, 1 out]
              "ADC value" <- w805
              n557 = Number To Decimal String(number=w854) -> (decimal integer string=w850:string)  [unwired: 1 in]
              n558 = Number To Decimal String(number=w834) -> (decimal integer string=w832:string)  [unwired: 1 in]
              n559 = String Length(string=w832) -> (length=w830:i32)
              n560 = Reverse String(1:w832) -> (0:w826:string)
              n561 = Reverse String(1:w850) -> (0:w851:string)
              n562 = Add(x=8.0, y=w809) -> (x+y=w820:dbl)
              n563 = Subtract(x=w811, y=8.0) -> (x-y=w818:dbl)
              n564 = Add(x=8.0, y=w810) -> (x+y=w819:dbl)
              n565 = case shown="1, Default" w830 {
                tunnel: ["00" "0" ""] -> w831
                frame 1, Default {
                }
                frame 2 {
                }
                frame 3 {
                }
              }
              n566 = local read "refnum out"() -> (w814:refnum<file>)
              n567 = In Range and Coerce(upper limit=w820, x=w805, lower limit=w809) -> (In Range?=w803:bool)  [unwired: 1 out]
              n568 = In Range and Coerce(upper limit=w811, x=w805, lower limit=w818) -> (In Range?=w801:bool)  [unwired: 1 out]
              n569 = In Range and Coerce(upper limit=w819, x=w805, lower limit=w810) -> (In Range?=w802:bool)  [unwired: 1 out]
              n570 = Search/Split String(string=w826, offset (0)=2) -> (substring before match=w827:string)  [unwired: 1 in, 2 out]
              n571 = Search/Split String(string=w851, offset (0)=1) -> (substring before match=w848:string)  [unwired: 1 in, 2 out]
              n572 = Search/Split String(string=w850, offset (0)=1) -> (substring before match=w847:string)  [unwired: 1 in, 2 out]
              n573 = case shown="True" w803 {
                tunnel: [w879 w887] -> w838
                tunnel: [w878 w886] -> w837
                tunnel: w814 -> [w879 w884]
                tunnel: w813 -> [w878 w883]
                tunnel: w805 -> [_ w882]
                frame False {
                }
                frame True {
                  n574 = Number To Fractional String(number=w882, precision (6)=i16 0) -> (F-format string=w888:string)  [unwired: 2 in]
                  n575 = Wait (ms)(milliseconds to wait=u32 50) -> ()  [unwired: 1 out]
                  n576 = call "dataSampled.vi"("Error In"=w883, "Data"=w888, "refnum in"=w884) -> ("error out"=w886:errorcluster, "refnum out"=w887:refnum<file>)  [unwired: 7 in]
                  "ADC low" <- TRUE
                }
              }
              n577 = Reverse String(1:w827) -> (0:w829:string)
              n578 = Concatenate Strings(w848, "." ("string"), w847) -> (w846:string)
              n579 = Concatenate Strings(w831, w832) -> (w833:string)
              n580 = Fract/Exp String To Number(string=w846) -> (number=w845:dbl)  [unwired: 3 in, 1 out]
              n581 = Search/Split String(string=w833, offset (0)=1) -> (substring before match=w828:string)  [unwired: 1 in, 2 out]
              n582 = case shown="True" w802 {
                tunnel: w838 -> [w868 w877]
                tunnel: w837 -> [w867 w876]
                tunnel: [w868 w874] -> w836
                tunnel: [w867 w873] -> w835
                tunnel: w805 -> [_ w871]
                frame False {
                }
                frame True {
                  n583 = Number To Fractional String(number=w871, precision (6)=i16 0) -> (F-format string=w875:string)  [unwired: 2 in]
                  n584 = Wait (ms)(milliseconds to wait=u32 50) -> ()  [unwired: 1 out]
                  n585 = call "dataSampled.vi"("Error In"=w876, "Data"=w875, "refnum in"=w877) -> ("error out"=w873:errorcluster, "refnum out"=w874:refnum<file>)  [unwired: 7 in]
                  "ADC mid" <- TRUE
                }
              }
              n586 = Concatenate Strings(w828, "." ("string"), w829) -> (w821:string)
              "current#" <- w821
              n587 = local read "ADC mid"() -> (w797:bool)
              n588 = local read "ADC low"() -> (w798:bool)
              n589 = local read "ADC hi"() -> (w796:bool)
              n590 = Fract/Exp String To Number(string=w821) -> (number=w815:dbl)  [unwired: 3 in, 1 out]
              n591 = Compound Arithmetic op=AND(w798, w797, w796) -> (w795:bool)
              "resistance result" <- w795
              n592 = case shown="True" w801 {
                tunnel: w836 -> [_ w866]
                tunnel: w835 -> [w859 w865]
                tunnel: [w859 w863] -> _
                tunnel: w805 -> [_ w862]
                frame False {
                }
                frame True {
                  n593 = Number To Fractional String(number=w862, precision (6)=i16 0) -> (F-format string=w864:string)  [unwired: 2 in]
                  n594 = call "dataSampled.vi"("Error In"=w865, "Data"=w864, "refnum in"=w866) -> ("error out"=w863:errorcluster)  [unwired: 7 in, 1 out]
                  "ADC hi" <- TRUE
                }
              }
              n595 = Less?(x=w815, y=w845) -> (x < y?=w799:bool)
              "overCurrent" <- w799
              n596 = Bundle(w805, w815) -> (→"RESISTANCE/CURRENT":cluster{dbl, dbl})  [unwired: 1 in]
              n597 = Or(x=w799, y="RES1") -> (x .or. y?=w800:bool)
              n598 = Not(x=w795) -> (.not. x?=w794:bool)
              n599 = Compound Arithmetic op=OR(w795, w800) -> (w839:bool)
              n600 = Compound Arithmetic op=AND(w794, w800) -> (w840:bool)
              n601 = Not(x=w840) -> (.not. x?=w793:bool)
            }
          }
        }
        n602 = Select(t=T1."Incline" ("Tab Control"), s=w762, f=T1."Failed" ("Tab Control")) -> (s? t:f=w765:T1)
      }
      frame "Pulse" {
        w898 = FALSE
        n603 = local write "BLE PULSE"(u32 0 ("Waveform Chart")) -> ()
        n604 = property on="BLE PULSE" class="WFChart (strict)"("History Data"=u32[] []) -> ()  [unwired: 2 in, 2 out]
        n605 = local write "PUL0"(w898) -> ()
        n606 = local write "PUL1"(w898) -> ()
        n607 = local read "EQF1259 com port"() -> (w896:refnum<visa-resource-name>)
        n608 = call "usbUart.vi"("VISA resource name"=w896, "write buffer"="h\u0001") -> ("byte[0]"=w894:string, "PartNumber"=w893:string)  [unwired: 2 in, 14 out]
        n609 = global write "Global_usbComm.vi" "PulseType"(w893) -> ()
        n610 = Not Equal?(x=w894, y="1") -> (x != y?=w900:bool)
        n611 = case shown="True" w900 {
          tunnel: [TRUE w910] -> w899
          frame False {
            n612 = local read "refnum out"() -> (w905:refnum<file>)
            n613 = call "dataSampled.vi"("refnum in"=w905) -> ()  [unwired: 9 in, 2 out]
          }
          frame True {
            n614 = call "pulsePIP.vi"() -> ("error out"=w906:errorcluster, "PULSE-17"=→"PULSE-17":string)  [unwired: 10 in]
            n615 = while {
              tunnel: [w917] -> w910
              tunnel: [w912] -> w908
              tunnel: w906 -> [w911]
              stop <- w916 stop-if-true
              n616 = local read "EQF1259 com port"() -> (w920:refnum<visa-resource-name>)
              n617 = Not(x="PUL1") -> (.not. x?=w915:bool)
              n618 = call "usbUart.vi"("VISA resource name"=w920, "write buffer"="F\u0001", "error in (no error)"=w911) -> ("number[0]"=→"BLE PULSE" →"Pulse#":u32, "error out"=w912:errorcluster)  [unwired: 1 in, 14 out]
              n619 = Compound Arithmetic op=OR("PUL0", "PUL1") -> (w916:bool)
              n620 = Compound Arithmetic op=AND("PUL0", w915) -> (w917:bool)
            }
            n621 = local read "refnum out"() -> (w909:refnum<file>)
            n622 = call "Pass_Fail.vi"("error in (no error)"=w908, "OK"=w910, "Byte Stream File in"=w909) -> ()  [unwired: 7 in, 2 out]
          }
        }
        n623 = Select(t=T1."Fan" ("Tab Control"), s=w899, f=T1."Failed" ("Tab Control")) -> (s? t:f=w901:T1)
      }
      frame "Fan" {
        w938 = FALSE
        n624 = local write "FanCurrent"(0.0 ("CURRENT")) -> ()
        n625 = property on="FanCurrent" class="WFChart (strict)"("History Data"=dbl[] []) -> ()  [unwired: 2 in, 2 out]
        n626 = local write "FAN0"(w938) -> ()
        n627 = local write "FAN1"(w938) -> ()
        n628 = local write "limitFan"(w938) -> ()
        n629 = flat-sequence {
          tunnel: [w944] -> w930
          tunnel: [w943] -> w929
          tunnel: w930 -> [w950]
          tunnel: [w950] -> w928
          tunnel: w929 -> [w949]
          tunnel: [w949] -> w926
          tunnel: [w946] -> w923
          tunnel: w928 -> [w955]
          tunnel: [w955] -> w927
          tunnel: w926 -> [w954]
          tunnel: [w953] -> w925
          tunnel: [w952] -> w924
          tunnel: w923 -> [w952]
          tunnel: w927 -> [w963]
          tunnel: [w963] -> w933
          tunnel: w925 -> [w962]
          tunnel: [w962] -> w932
          tunnel: [w959] -> w931
          tunnel: w924 -> [w957]
          tunnel: w933 -> [w971]
          tunnel: w932 -> [w966]
          tunnel: [w965] -> w935
          tunnel: [w964] -> w934
          tunnel: w931 -> [w964]
          frame #0 {
            n630 = local read "EQF1259 com port"() -> (w944:refnum<visa-resource-name>)
            n631 = call "usbUart.vi"("VISA resource name"=w944, "write buffer"="P\u0002") -> ("error out"=w943:errorcluster)  [unwired: 2 in, 15 out]
          }
          frame #1 {
            n632 = global read "Global_usbComm.vi" "FAN"() -> (w948:string)
            "FAN" <- w948
            n633 = Not Equal?(x=w948, y="0") -> (x != y?=w946:bool)
          }
          frame #2 {
            n634 = call "usbUart.vi"("VISA resource name"=w955, "write buffer"="b\u0001", "error in (no error)"=w954) -> ("binary[0] String"=w951:string, "error out"=w953:errorcluster)  [unwired: 1 in, 14 out]
            n635 = global write "Global_usbComm.vi" "fanType"(w951) -> ()
          }
          frame #3 {
            n636 = global read "Global_usbComm.vi" "fanType"() -> (w961:string)
            "fanType" <- w961
            n637 = Not Equal?(x=w961, y="0") -> (x != y?=w958:bool)
            n638 = And(x=w958, y=w957) -> (x .and. y?=w959:bool)
          }
          frame #4 {
            n639 = call "usbUart.vi"("VISA resource name"=w971, "write buffer"="p\u0001", "error in (no error)"=w966) -> ("number[0]"=w975:u32, "error out"=w965:errorcluster)  [unwired: 1 in, 14 out]
            n640 = Number To Decimal String(number=w975) -> (decimal integer string=w973:string)  [unwired: 1 in]
            n641 = Reverse String(1:w973) -> (0:w974:string)
            n642 = Search/Split String(string=w973, offset (0)=1) -> (substring before match=w976:string)  [unwired: 1 in, 2 out]
            n643 = Search/Split String(string=w974, offset (0)=1) -> (substring before match=w977:string)  [unwired: 1 in, 2 out]
            n644 = Concatenate Strings(w976, "." ("string"), w977) -> (→"currentMaxFan":string)
          }
        }
        n645 = case shown="True" w934 {
          tunnel: [TRUE w984] -> w942
          tunnel: w935 -> [w978 w981]
          frame False {
            n646 = local read "refnum out"() -> (w980:refnum<file>)
            n647 = call "dataSampled.vi"("Error In"=w978, "refnum in"=w980) -> ()  [unwired: 8 in, 2 out]
          }
          frame True {
            n648 = while {
              tunnel: [w988] -> w984
              tunnel: [w991] -> w983
              tunnel: w981 -> [w985]
              stop <- w998 stop-if-true
              n649 = call "fanPIP.vi"("error in (no error)"=w985) -> ("error out"=w990:errorcluster, "FAN-18"=→"FAN-18":string)  [unwired: 9 in]
              n650 = local read "EQF1259 com port"() -> (w994:refnum<visa-resource-name>)
              n651 = local read "currentMaxFan"() -> (w993:string)
              n652 = call "currentScan.vi"("error in (no error)"=w990, "Imax"=w993, "VISA resource name"=w994) -> ("max"=w992:bool, "Istring"=w991:string, "Ichart"=→"FanCurrent":dbl)  [unwired: 5 in, 1 out]
              "Ifan" <- w991
              "limitFan" <- w992
              n653 = Not(x="FAN1") -> (.not. x?=w987:bool)
              n654 = Compound Arithmetic op=OR("FAN0", "FAN1", w992) -> (w998:bool)
              n655 = Not(x=w992) -> (.not. x?=w986:bool)
              n656 = Compound Arithmetic op=AND("FAN0", w987, w986) -> (w988:bool)
            }
            n657 = local read "refnum out"() -> (w982:refnum<file>)
            n658 = call "dataSampled.vi"("Data"=w983, "refnum in"=w982) -> ()  [unwired: 8 in, 2 out]
          }
        }
        n659 = Select(t=T1."Audio" ("Tab Control"), s=w942, f=T1."Failed" ("Tab Control")) -> (s? t:f=w941:T1)
      }
      frame "Audio" {
        w1019 = FALSE
        n660 = property on="AudioCurrent" class="WFChart (strict)"("History Data"=dbl[] []) -> ()  [unwired: 2 in, 2 out]
        n661 = local write "AUD1"(w1019) -> ()
        n662 = local write "AUD0"(w1019) -> ()
        n663 = local write "limitAudio"(w1019) -> ()
        n664 = local read "EQF1259 com port"() -> (w1011:refnum<visa-resource-name>)
        n665 = call "usbUart.vi"("VISA resource name"=w1011, "write buffer"="`\u0002") -> ("PartNumber"=w1002:string, "number[0]"=w1006:u32)  [unwired: 2 in, 14 out]
        n666 = call "usbUart.vi"("VISA resource name"=w1011, "write buffer"="p\u0001") -> ("number[0]"=w1009:u32)  [unwired: 2 in, 15 out]
        n667 = Number To Decimal String(number=w1006) -> (decimal integer string=w1005:string)  [unwired: 1 in]
        n668 = Number To Decimal String(number=w1009) -> (decimal integer string=w1012:string)  [unwired: 1 in]
        n669 = Not Equal?(x=w1002, y="1") -> (x != y?=w1022:bool)
        n670 = global write "Global_usbComm.vi" "AudioType"(w1005) -> ()
        n671 = case shown="True" w1022 {
          tunnel: [TRUE w1028] -> w1021
          frame False {
            n672 = local read "refnum out"() -> (w1024:refnum<file>)
            n673 = call "dataSampled.vi"("refnum in"=w1024) -> ()  [unwired: 9 in, 2 out]
          }
          frame True {
            n674 = while {
              tunnel: [w1040] -> w1028
              tunnel: [w1033] -> w1026
              stop <- w1041 stop-if-true
              n675 = local read "EQF1259 com port"() -> (w1038:refnum<visa-resource-name>)
              n676 = local read "currentMaxAudio"() -> (w1037:string)
              n677 = call "audio_tvPIP.vi"() -> ("error out"=w1029:errorcluster, "AUDIO-19"=→"AUDIO-19":string)  [unwired: 9 in, 1 out]
              n678 = call "currentScan.vi"("error in (no error)"=w1029, "Imax"=w1037, "VISA resource name"=w1038) -> ("max"=w1036:bool, "Istring"=w1033:string, "Ichart"=→"AudioCurrent":dbl)  [unwired: 5 in, 1 out]
              "Iaudio" <- w1033
              "limitAudio" <- w1036
              n679 = Compound Arithmetic op=OR("AUD0", "AUD1", w1036) -> (w1041:bool)
              n680 = Not(x="AUD0") -> (.not. x?=w1034:bool)
              n681 = Not(x=w1036) -> (.not. x?=w1035:bool)
              n682 = Compound Arithmetic op=AND(w1034, "AUD1", w1035) -> (w1040:bool)
            }
            n683 = local read "refnum out"() -> (w1027:refnum<file>)
            n684 = call "dataSampled.vi"("Data"=w1026, "refnum in"=w1027) -> ()  [unwired: 8 in, 2 out]
          }
        }
        n685 = Reverse String(1:w1012) -> (0:w1016:string)
        n686 = Search/Split String(string=w1012, offset (0)=1) -> (substring before match=w1007:string)  [unwired: 1 in, 2 out]
        n687 = Search/Split String(string=w1016, offset (0)=1) -> (substring before match=w1008:string)  [unwired: 1 in, 2 out]
        n688 = Concatenate Strings(w1007, "." ("string"), w1008) -> (→"currentMaxAudio":string)
        n689 = Select(t=T1."TV" ("Tab Control"), s=w1021, f=T1."Failed" ("Tab Control")) -> (s? t:f=w1023:T1)
      }
      frame "TV" {
        w1050 = FALSE
        n690 = local write "TV0"(w1050) -> ()
        n691 = local write "TV1"(w1050) -> ()
        n692 = property on="TVCurrent" class="WFChart (strict)"("History Data"=dbl[] []) -> ()  [unwired: 2 in, 2 out]
        n693 = local write "limitTV"(w1050) -> ()
        n694 = while {
          shift-right: [w1056] -> _
          shift-left: 0 -> [w1057]
          tunnel: [w1055] -> w1044
          tunnel: [w1054] -> w1045
          stop <- w1053 stop-if-true
          n695 = case shown="4" w1057 {
            tunnel: [1 2 3 4 _] -> w1056
            tunnel: [w1060 w1074 w1083 w1091 _] -> w1055
            tunnel: [FALSE _ _ _ w1099] -> w1054
            tunnel: [FALSE _ _ _ TRUE] -> w1053
            frame 0, Default {
              n696 = local read "EQF1259 com port"() -> (w1072:refnum<visa-resource-name>)
              n697 = call "usbUart.vi"("VISA resource name"=w1072, "write buffer"="p\u0001") -> ("number[0]"=w1071:u32, "error out"=w1060:errorcluster)  [unwired: 2 in, 14 out]
              n698 = Number To Decimal String(number=w1071) -> (decimal integer string=w1067:string)  [unwired: 1 in]
              n699 = Reverse String(1:w1067) -> (0:w1066:string)
              n700 = Search/Split String(string=w1067, offset (0)=1) -> (substring before match=w1069:string)  [unwired: 1 in, 2 out]
              n701 = Search/Split String(string=w1066, offset (0)=1) -> (substring before match=w1070:string)  [unwired: 1 in, 2 out]
              n702 = Concatenate Strings(w1069, "." ("string"), w1070) -> (→"currentMaxTV":string)
            }
            frame 1 {
              n703 = flat-sequence {
                tunnel: [w1077] -> w1073
                tunnel: [w1079] -> w1074
                tunnel: w1073 -> [w1079]
                frame #0 {
                  n704 = local read "EQF1259 com port"() -> (w1076:refnum<visa-resource-name>)
                  n705 = call "usbUart.vi"("VISA resource name"=w1076, "write buffer"="S\u0002") -> ("error out"=w1077:errorcluster)  [unwired: 2 in, 15 out]
                }
                frame #1 {
                  n706 = global read "Global_usbComm.vi" "TV"() -> (→"TV":string)
                  n707 = global read "Global_usbComm.vi" "Display"() -> (→"Display")
                }
              }
            }
            frame 2 {
              n708 = flat-sequence {
                tunnel: [w1086] -> w1082
                tunnel: [w1088] -> w1083
                tunnel: w1082 -> [w1088]
                frame #0 {
                  n709 = local read "EQF1259 com port"() -> (w1085:refnum<visa-resource-name>)
                  n710 = call "usbUart.vi"("VISA resource name"=w1085, "write buffer"="S\u0002") -> ("error out"=w1086:errorcluster)  [unwired: 2 in, 15 out]
                }
                frame #1 {
                  n711 = global read "Global_usbComm.vi" "AudioType"() -> (→"audioType")
                }
              }
            }
            frame 3 {
              n712 = flat-sequence {
                tunnel: [w1094] -> w1091
                frame #0 {
                  n713 = local read "EQF1259 com port"() -> (w1093:refnum<visa-resource-name>)
                  n714 = call "usbUart.vi"("VISA resource name"=w1093, "write buffer"="š\u0001") -> ("PartNumber"=→"tabletType":string, "error out"=w1094:errorcluster)  [unwired: 2 in, 14 out]
                }
              }
            }
            frame 4 {
              w1102 = 128
              n715 = global read "Global_usbComm.vi" "AudioType"() -> (w1105)
              n716 = local read "TV"() -> (w1108:string)
              n717 = Decimal String To Number(string=w1105) -> (number=w1103:i32)  [unwired: 2 in, 1 out]
              n718 = Decimal String To Number(string=w1108) -> (number=w1104:i32)  [unwired: 2 in, 1 out]
              n719 = local read "tabletType"() -> (w1098:string)
              n720 = Greater Or Equal?(x=w1104, y=w1102) -> (x >= y?=w1107:bool)
              n721 = Greater Or Equal?(x=w1103, y=w1102) -> (x >= y?=w1106:bool)
              n722 = Compound Arithmetic op=OR(w1107, w1106) -> (w1101:bool)
              n723 = Equal?(x="1", y=w1098) -> (x = y?=w1096:bool)
              n724 = Or(x=w1096, y=w1101) -> (x .or. y?=w1099:bool)
            }
          }
        }
        n725 = case shown="True" w1045 {
          tunnel: [TRUE w1114] -> w1052
          tunnel: w1044 -> [_ w1111]
          frame False {
            n726 = local read "refnum out"() -> (w1109:refnum<file>)
            n727 = call "dataSampled.vi"("refnum in"=w1109) -> ()  [unwired: 9 in, 2 out]
          }
          frame True {
            n728 = while {
              tunnel: [w1130] -> w1114
              tunnel: [w1122] -> w1112
              tunnel: w1111 -> [w1115]
              stop <- w1131 stop-if-true
              n729 = local read "tabletType"() -> (w1116:string)
              n730 = Equal?(x=w1116, y="1") -> (x = y?=w1119:bool)
              n731 = case shown="True" w1119 {
                tunnel: [w1134 w1136] -> w1121
                tunnel: [w1133 _] -> w1118
                tunnel: w1115 -> [w1132 _]
                frame False {
                  n732 = call "audio_tvPIP.vi"("error in (no error)"=w1132) -> ("error out"=w1133:errorcluster, "TV-20"=w1134:string)  [unwired: 8 in, 1 out]
                }
                frame True {
                  n733 = global read "Global_usbComm.vi" "PIP_Instruction"() -> (w1135:string[][])
                  n734 = Index Array(array=w1135, index (row)=1 ("disabled index (row)"), index (col)=20 ("disabled index (col)")) -> (element=w1136:string)
                }
              }
              "TV-20" <- w1121
              n735 = local read "EQF1259 com port"() -> (w1126:refnum<visa-resource-name>)
              n736 = local read "currentMaxTV"() -> (w1125:string)
              n737 = call "currentScan.vi"("error in (no error)"=w1118, "Imax"=w1125, "VISA resource name"=w1126) -> ("max"=w1123:bool, "Istring"=w1122:string, "Ichart"=→"TVCurrent":dbl)  [unwired: 5 in, 1 out]
              "Itv" <- w1122
              "limitTV" <- w1123
              n738 = Not(x="TV1") -> (.not. x?=w1117:bool)
              n739 = Compound Arithmetic op=OR("TV1", "TV0", w1123) -> (w1131:bool)
              n740 = Not(x=w1123) -> (.not. x?=w1124:bool)
              n741 = Compound Arithmetic op=AND(w1117, "TV0", w1124) -> (w1130:bool)
            }
            n742 = local read "refnum out"() -> (w1113:refnum<file>)
            n743 = call "dataSampled.vi"("Data"=w1112, "refnum in"=w1113) -> ()  [unwired: 8 in, 2 out]
          }
        }
        n744 = Select(t=T1."USB" ("Tab Control"), s=w1052, f=T1."Failed" ("Tab Control")) -> (s? t:f=w1051:T1)
      }
      frame "USB" {
        w1149 = FALSE
        n745 = local write "FanCurrent"(0.0 ("CURRENT")) -> ()
        n746 = property on="FanCurrent" class="WFChart (strict)"("History Data"=dbl[] []) -> ()  [unwired: 2 in, 2 out]
        n747 = local write "USB0"(w1149) -> ()
        n748 = local write "USB1"(w1149) -> ()
        n749 = local write "limitUSB"(w1149) -> ()
        n750 = local read "EQF1259 com port"() -> (w1148:refnum<visa-resource-name>)
        n751 = flat-sequence {
          tunnel: [w1154] -> w1146
          tunnel: w1148 -> [w1153]
          tunnel: [w1153] -> w1144
          tunnel: w1146 -> [w1159]
          tunnel: [w1159] -> w1145
          tunnel: w1144 -> [w1158]
          tunnel: [w1158] -> w1143
          tunnel: w1145 -> [w1164]
          tunnel: w1143 -> [w1160]
          tunnel: [w1175] -> w1147
          frame #0 {
            n752 = call "usbUart.vi"("VISA resource name"=w1153, "write buffer"="S\u0002") -> ("error out"=w1154:errorcluster)  [unwired: 2 in, 15 out]
          }
          frame #1 {
            n753 = global read "Global_usbComm.vi" "TABLET"() -> (w1156:string)
            n754 = local write "tabletType"(w1156) -> ()
            n755 = global read "Global_usbComm.vi" "USB"() -> (→"USB":string)
          }
          frame #2 {
            n756 = call "usbUart.vi"("VISA resource name"=w1160, "write buffer"="p\u0001", "error in (no error)"=w1164) -> ("number[0]"=w1171:u32)  [unwired: 1 in, 15 out]
            n757 = Number To Decimal String(number=w1171) -> (decimal integer string=w1167:string)  [unwired: 1 in]
            n758 = Reverse String(1:w1167) -> (0:w1166:string)
            n759 = Search/Split String(string=w1167, offset (0)=1) -> (substring before match=w1169:string)  [unwired: 1 in, 2 out]
            n760 = Search/Split String(string=w1166, offset (0)=1) -> (substring before match=w1170:string)  [unwired: 1 in, 2 out]
            n761 = Concatenate Strings(w1169, "." ("string"), w1170) -> (→"currentMaxUSB":string)
          }
          frame #3 {
            n762 = local read "tabletType"() -> (w1172:string)
            n763 = Equal?(x=w1172, y="1") -> (x = y?=w1174:bool)
            n764 = case shown="True" w1174 {
              tunnel: [FALSE TRUE] -> w1173
              frame False {
                # "usb is enabled on Arogon"
              }
              frame True {
              }
            }
            n765 = case shown="True" w1173 {
              tunnel: [TRUE w1183] -> w1175
              frame False {
                n766 = local read "refnum out"() -> (w1179:refnum<file>)
                n767 = call "dataSampled.vi"("refnum in"=w1179) -> ()  [unwired: 9 in, 2 out]
              }
              frame True {
                n768 = while {
                  tunnel: [w1209] -> w1183
                  tunnel: [w1194] -> w1181
                  stop <- w1212 stop-if-true
                  n769 = local read "EQF1259 com port"() -> (w1190:refnum<visa-resource-name>)
                  n770 = global read "Global_usbComm.vi" "PIP_Instruction"() -> (w1187:string[][])
                  n771 = Index Array(array=w1187, index (row)=1 ("disabled index (row)"), index (col)=16 ("disabled index (col)")) -> (element=→"USB-16":string)
                  n772 = call "usbUart.vi"("VISA resource name"=w1190, "write buffer"="n\u0002") -> ("number[0]"=w1208:u32)  [unwired: 2 in, 15 out]
                  n773 = Number To Decimal String(number=w1208) -> (decimal integer string=w1206:string)  [unwired: 1 in]
                  n774 = String Length(string=w1206) -> (length=w1204:i32)
                  n775 = Reverse String(1:w1206) -> (0:w1200:string)
                  n776 = case shown="1, Default" w1204 {
                    tunnel: ["00" "0" ""] -> w1205
                    frame 1, Default {
                    }
                    frame 2 {
                    }
                    frame 3 {
                    }
                  }
                  n777 = Search/Split String(string=w1200, offset (0)=2) -> (substring before match=w1201:string)  [unwired: 1 in, 2 out]
                  n778 = Reverse String(1:w1201) -> (0:w1203:string)
                  n779 = Concatenate Strings(w1205, w1206) -> (w1207:string)
                  n780 = Search/Split String(string=w1207, offset (0)=1) -> (substring before match=w1202:string)  [unwired: 1 in, 2 out]
                  n781 = Concatenate Strings(w1202, "." ("string"), w1203) -> (w1194:string)
                  "Iusb" <- w1194
                  n782 = local read "currentMaxUSB"() -> (w1195:string)
                  n783 = Fract/Exp String To Number(string=w1195) -> (number=w1193:dbl)  [unwired: 3 in, 1 out]
                  n784 = Fract/Exp String To Number(string=w1194) -> (number=→"USBCurrent":dbl)  [unwired: 3 in, 1 out]
                  n785 = Fract/Exp String To Number(string=w1194) -> (number=w1192:dbl)  [unwired: 3 in, 1 out]
                  n786 = Equal?(x=w1193, y=w1192) -> (x = y?=w1191:bool)
                  "limitUSB" <- w1191
                  n787 = Compound Arithmetic op=OR("USB0", "USB1", w1191) -> (w1212:bool)
                  n788 = Not(x="USB1") -> (.not. x?=w1213:bool)
                  n789 = Not(x=w1191) -> (.not. x?=w1188:bool)
                  n790 = Compound Arithmetic op=AND("USB0", w1213, w1188) -> (w1209:bool)
                }
                n791 = local read "refnum out"() -> (w1182:refnum<file>)
                n792 = call "dataSampled.vi"("Data"=w1181, "refnum in"=w1182) -> ()  [unwired: 8 in, 2 out]
              }
            }
          }
        }
        n793 = Select(t=T1."Resistance" ("Tab Control"), s=w1147, f=T1."Failed" ("Tab Control")) -> (s? t:f=w1151:T1)
      }
      frame "CSafe" {
        w1225 = FALSE
        n794 = local write "FanCurrent"(0.0 ("CURRENT")) -> ()
        n795 = property on="FanCurrent" class="WFChart (strict)"("History Data"=dbl[] []) -> ()  [unwired: 2 in, 2 out]
        n796 = local write "CSA0"(w1225) -> ()
        n797 = local write "CSA1"(w1225) -> ()
        n798 = local read "EQF1259 com port"() -> (w1231:refnum<visa-resource-name>)
        n799 = local write "limitCSafe"(w1225) -> ()
        n800 = call "usbUart.vi"("VISA resource name"=w1231, "write buffer"="P\u0002") -> ()  [unwired: 2 in, 16 out]
        n801 = call "usbUart.vi"("VISA resource name"=w1231, "write buffer"="p\u0001") -> ("number[0]"=w1222:u32)  [unwired: 2 in, 15 out]
        n802 = Number To Decimal String(number=w1222) -> (decimal integer string=w1233:string)  [unwired: 1 in]
        n803 = Reverse String(1:w1233) -> (0:w1234:string)
        n804 = Search/Split String(string=w1233, offset (0)=1) -> (substring before match=w1223:string)  [unwired: 1 in, 2 out]
        n805 = Search/Split String(string=w1234, offset (0)=1) -> (substring before match=w1224:string)  [unwired: 1 in, 2 out]
        n806 = Concatenate Strings(w1223, "." ("string"), w1224) -> (→"currentMaxCSafe":string)
        n807 = global read "Global_usbComm.vi" "CSAFE"() -> (w1221:string)
        n808 = Not Equal?(x=w1221, y="0") -> (x != y?=w1229:bool)
        n809 = case shown="False" w1229 {
          tunnel: [TRUE w1245] -> w1240
          frame False {
            n810 = local read "refnum out"() -> (w1241:refnum<file>)
            n811 = call "dataSampled.vi"("refnum in"=w1241) -> ()  [unwired: 9 in, 2 out]
          }
          frame True {
            n812 = while {
              tunnel: [w1268] -> w1245
              tunnel: [w1253] -> w1243
              stop <- w1271 stop-if-true
              n813 = local read "EQF1259 com port"() -> (w1249:refnum<visa-resource-name>)
              n814 = call "csafePIP.vi"() -> ("error out"=w1247:errorcluster, "CSAFE-21"=→"CSAFE-21":string)  [unwired: 10 in]
              n815 = call "usbUart.vi"("VISA resource name"=w1249, "write buffer"="n\u0002", "error in (no error)"=w1247) -> ("number[0]"=w1267:u32)  [unwired: 1 in, 15 out]
              n816 = Number To Decimal String(number=w1267) -> (decimal integer string=w1265:string)  [unwired: 1 in]
              n817 = String Length(string=w1265) -> (length=w1263:i32)
              n818 = Reverse String(1:w1265) -> (0:w1259:string)
              n819 = case shown="1, Default" w1263 {
                tunnel: ["00" "0" ""] -> w1264
                frame 1, Default {
                }
                frame 2 {
                }
                frame 3 {
                }
              }
              n820 = Search/Split String(string=w1259, offset (0)=2) -> (substring before match=w1260:string)  [unwired: 1 in, 2 out]
              n821 = Reverse String(1:w1260) -> (0:w1262:string)
              n822 = Concatenate Strings(w1264, w1265) -> (w1266:string)
              n823 = Search/Split String(string=w1266, offset (0)=1) -> (substring before match=w1261:string)  [unwired: 1 in, 2 out]
              n824 = Concatenate Strings(w1261, "." ("string"), w1262) -> (w1253:string)
              "Icsafe" <- w1253
              n825 = local read "currentMaxCSafe"() -> (w1254:string)
              n826 = Fract/Exp String To Number(string=w1254) -> (number=w1252:dbl)  [unwired: 3 in, 1 out]
              n827 = Fract/Exp String To Number(string=w1253) -> (number=→"CSafeCurrent":dbl)  [unwired: 3 in, 1 out]
              n828 = Fract/Exp String To Number(string=w1253) -> (number=w1251:dbl)  [unwired: 3 in, 1 out]
              n829 = Not(x="CSA1") -> (.not. x?=w1272:bool)
              n830 = Equal?(x=w1252, y=w1251) -> (x = y?=w1250:bool)
              "limitCSafe" <- w1250
              n831 = Compound Arithmetic op=AND("CSA0", w1272, w1250) -> (w1268:bool)
              n832 = Compound Arithmetic op=OR("CSA0", "CSA1", w1250) -> (w1271:bool)
            }
            n833 = local read "refnum out"() -> (w1244:refnum<file>)
            n834 = call "dataSampled.vi"("Data"=w1243, "refnum in"=w1244) -> ()  [unwired: 8 in, 2 out]
          }
        }
        n835 = Select(t=T1."Wahoo" ("Tab Control"), s=w1240, f=T1."Failed" ("Tab Control")) -> (s? t:f=w1228:T1)
      }
      frame "Wahoo" {
        w1282 = FALSE
        n836 = local write "FanCurrent"(0.0 ("CURRENT")) -> ()
        n837 = property on="FanCurrent" class="WFChart (strict)"("History Data"=dbl[] []) -> ()  [unwired: 2 in, 2 out]
        n838 = local write "WAH0"(w1282) -> ()
        n839 = local write "WAH1"(w1282) -> ()
        n840 = local read "EQF1259 com port"() -> (w1285:refnum<visa-resource-name>)
        n841 = local write "limitWahoo"(w1282) -> ()
        n842 = call "usbUart.vi"("VISA resource name"=w1285, "write buffer"="P\u0002") -> ()  [unwired: 2 in, 16 out]
        n843 = call "usbUart.vi"("VISA resource name"=w1285, "write buffer"="p\u0001") -> ("number[1]"=w1296:u32)  [unwired: 2 in, 15 out]
        n844 = Number To Decimal String(number=w1296) -> (decimal integer string=w1292:string)  [unwired: 1 in]
        n845 = Reverse String(1:w1292) -> (0:w1293:string)
        n846 = Search/Split String(string=w1292, offset (0)=1) -> (substring before match=w1289:string)  [unwired: 1 in, 2 out]
        n847 = Search/Split String(string=w1293, offset (0)=1) -> (substring before match=w1290:string)  [unwired: 1 in, 2 out]
        n848 = Concatenate Strings(w1290, "." ("string"), w1289) -> (→"currentMaxWahoo":string)
        n849 = global read "Global_usbComm.vi" "WAHOO"() -> (w1281:string)
        n850 = Not Equal?(x=w1281, y="0" ("WAHOO")) -> (x != y?=w1286:bool)
        n851 = case shown="True" w1286 {
          tunnel: [TRUE w1304] -> w1280
          frame False {
            n852 = local read "refnum out"() -> (w1300:refnum<file>)
            n853 = call "dataSampled.vi"("refnum in"=w1300) -> ()  [unwired: 9 in, 2 out]
          }
          frame True {
            n854 = while {
              tunnel: [w1327] -> w1304
              tunnel: [w1312] -> w1303
              stop <- w1330 stop-if-true
              n855 = local read "EQF1259 com port"() -> (w1308:refnum<visa-resource-name>)
              n856 = call "wahooPIP.vi"() -> ("error out"=w1306:errorcluster, "WAHOO-22"=→"WAHOO-22":string)  [unwired: 10 in]
              n857 = call "usbUart.vi"("VISA resource name"=w1308, "write buffer"="n\u0002", "error in (no error)"=w1306) -> ("number[0]"=w1326:u32)  [unwired: 1 in, 15 out]
              n858 = Number To Decimal String(number=w1326) -> (decimal integer string=w1324:string)  [unwired: 1 in]
              n859 = String Length(string=w1324) -> (length=w1322:i32)
              n860 = Reverse String(1:w1324) -> (0:w1318:string)
              n861 = case shown="1, Default" w1322 {
                tunnel: ["00" "0" ""] -> w1323
                frame 1, Default {
                }
                frame 2 {
                }
                frame 3 {
                }
              }
              n862 = Search/Split String(string=w1318, offset (0)=2) -> (substring before match=w1319:string)  [unwired: 1 in, 2 out]
              n863 = Reverse String(1:w1319) -> (0:w1321:string)
              n864 = Concatenate Strings(w1323, w1324) -> (w1325:string)
              n865 = Search/Split String(string=w1325, offset (0)=1) -> (substring before match=w1320:string)  [unwired: 1 in, 2 out]
              n866 = Concatenate Strings(w1320, "." ("string"), w1321) -> (w1312:string)
              "Iwahoo" <- w1312
              n867 = local read "currentMaxWahoo"() -> (w1313:string)
              n868 = Fract/Exp String To Number(string=w1313) -> (number=w1311:dbl)  [unwired: 3 in, 1 out]
              n869 = Fract/Exp String To Number(string=w1312) -> (number=→"WahooCurrent":dbl)  [unwired: 3 in, 1 out]
              n870 = Fract/Exp String To Number(string=w1312) -> (number=w1310:dbl)  [unwired: 3 in, 1 out]
              n871 = Not(x="WAH1") -> (.not. x?=w1331:bool)
              n872 = Equal?(x=w1311, y=w1310) -> (x = y?=w1309:bool)
              "limitWahoo" <- w1309
              n873 = Compound Arithmetic op=AND("WAH0", w1331, w1309) -> (w1327:bool)
              n874 = Compound Arithmetic op=OR("WAH0", "WAH1", w1309) -> (w1330:bool)
            }
            n875 = local read "refnum out"() -> (w1302:refnum<file>)
            n876 = call "dataSampled.vi"("Data"=w1303, "refnum in"=w1302) -> ()  [unwired: 8 in, 2 out]
          }
        }
        n877 = Select(t=T1."Another" ("Tab Control"), s=w1280, f=T1."Failed" ("Tab Control")) -> (s? t:f=w1288:T1)
      }
      frame "Another" {
        w1346 = FALSE
        n878 = local read "refnum out"() -> (w1345:refnum<file>)
        n879 = local write "ANO0"(w1346) -> ()
        n880 = local write "ANO1"(w1346) -> ()
        n881 = local read "EQF1259 com port"() -> (w1337:refnum<visa-resource-name>)
        n882 = Write to Text File(file (use dialog)=w1345, text="\r") -> ()  [unwired: 2 in, 3 out]
        n883 = call "usbUart.vi"("VISA resource name"=w1337, "write buffer"="(\u0001") -> ()  [unwired: 2 in, 16 out]
        n884 = call "JPG_import.vi"("File name"="smiley" ("Complete File path"), "File path"="C:\\specsheetsConsole\\Documentation\\" ("File name")) -> ("new picture"=→"Another":picture)  [unwired: 7 in, 2 out]
        n885 = while {
          tunnel: [w1349] -> w1348
          stop <- w1352 stop-if-true
          n886 = Compound Arithmetic op=OR("ANO1", "ANO0") -> (w1352:bool)
          n887 = Not(x="ANO0") -> (.not. x?=w1353:bool)
          n888 = Compound Arithmetic op=AND("ANO1", w1353) -> (w1349:bool)
        }
        n889 = Select(t=T1."Scan DUT" ("Tab Control"), s=w1348, f=T1."end" ("Tab Control")) -> (s? t:f=w1347:T1)
      }
      frame "Failed" {
        n890 = call "Display Message to User6"() -> ()  [unwired: 10 in, 2 out]
        n891 = Add(x=w1356, y=1) -> (x+y=w1355:i32)
        "# of Failed Samples" <- w1355
        n892 = local read "refnum out"() -> (w1364:refnum<file>)
        n893 = local read "EQF1259 com port"() -> (w1358:refnum<visa-resource-name>)
        n894 = call "dataSampled.vi"("Data"="Sample Failed" ("string"), "refnum in"=w1364) -> ()  [unwired: 8 in, 2 out]
        n895 = call "usbUart.vi"("VISA resource name"=w1358, "write buffer"="(\u0001") -> ()  [unwired: 2 in, 16 out]
        n896 = call "JPG_import.vi"("File name"="frowny" ("Complete File path"), "File path"="C:\\specsheetsConsole\\Documentation\\" ("File name")) -> ("new picture"=→"Failed":picture)  [unwired: 7 in, 2 out]
      }
      frame "end" {
        n897 = local read "refnum out"() -> (w1374:refnum<file>)
        n898 = call "Close Data File and open.vi"("File Refnum In"=w1374) -> ("error out"=w1373:errorcluster, "path"=w1375:path)  [unwired: 9 in]
        n899 = Path To String(path=w1375) -> (string=w1376:string)
        "Test Log" <- w1376
        n900 = call "CMD execution.vi"("Path"=w1376, "error in (no error)"=w1373) -> ()  [unwired: 13 in, 1 out]
        n901 = call "JPG_import.vi"("File name"="intro" ("Complete File path"), "File path"="C:\\specsheetsConsole\\Documentation\\" ("File name")) -> ("new picture"=→"Goodbye!":picture)  [unwired: 7 in, 2 out]
      }
    }
  }
